vi "SCMP - Main Program v3.vi"() -> ()   [LabVIEW 2014]
doc: "Goodrich Exposure Range: .05microseconds to 798.9ms\n\nLow Gain (110e-/ADU)\nHigh Gain (6.5 e-/ADU)\n\nGA1280J Trigger Modes\n0 : Internally triggered; Internally timed\n1 : Externally triggered; Internally timed\n2 : Externally triggered; Externally timed\n3 : Externally gated; Internally timed\n\nFor list of camera commands\nsee Appendix A in the manual\n\n\nUse this template to build a standard state machine design pattern. Each state executes code and determines which state to transition to. Contrast this design pattern with the User Interface Event Handler pattern, in which code executes in response to user actions. Contrast this design pattern also with the Queued Message Handler pattern, in which each message handling code can queue zero or more new messages.\nNote: This template does not contain the most recent programming guidelines recommended by National Instruments. For a complete, project-based implementation of the Standard State Machine pattern, use the Create Project dialog box instead of this template."
uses:
  Controls/Main Program States.ctl
  <vilib>/Utility/error.llb/DialogType.ctl
  Controls/SCD - Calibration Optics Filter Wheel.ctl
  Controls/SCD - EDT - Emission Line Filter Wheel.ctl
  Controls/CoMP-S Controls/Emission Line Filter Wheel.ctl
  Controls/CoMP-S Controls/Polarization Optics Filter Wheel.ctl
  Controls/Global demo.vi
  Controls/SCD - FITS Cluster.ctl
  AISAS/Controls/focus.ctl
  AISAS/Controls/Diffuser.ctl
  Controls/Globals.vi
  AISAS/Mech/AISAS Mech.lvclass
  c:/mhutar/SCMP/Ancillary/Watlow EZ-ZONE/Public/Watbus.dll
  Ancillary/Watlow EZ-ZONE/Public/Watbus.dll
  Controls/peripherals.ctl
  AISAS/Controls/motor.ctl
  Camera/Camera/Camera.lvclass
  Controls/Cameras select.ctl
  Camera/Andor Neo/Andor.lvclass
  Controls/FITS Data type.ctl
  Controls/Cbk Data type.ctl
  Controls/Cookbook.ctl
  Controls/beaning.ctl
  PI/PI Control.ctl
  AISAS/Controls/Rotation.ctl
panel:
  in  "Comment":string="Test"
  in  "Observer":string="Observer"
  out "Instrument":string
  out "Main Loop":bool=TRUE
  out "Log Loop":bool=TRUE
  out "Program":bool=TRUE
  out "Version":string
  in  "AOI Width 2":i64=2560
  in  "AOI Height 2":i64=2160
  out "Latest Actions":string="\r"
  out "cbk name":string="automated_find_focus_656.cbk"
  out "Main Loop Error":errorcluster={"status"=TRUE, "code"=0, "source"=""}
  in  "Tab Control":T1(tab)
  in  "Live Preview":bool
  in  "Snap Images":bool
  out "Camera T Image Zoom":u32[][](graph)
  out "Histogram Graph 2":T2(graph)
  out "Timestamp 2":timestamp=timestamp(3507746192.5616717 s since 1904-01-01)
  out "Mean ADU 2":u32=7788 format="%.1f"
  out "Sharpness 2":dbl format="%.2f"
  out "Camera FITS file path 2":path
  out "Camera R Image":u32[][](graph)
  in  "PI cam3 (mm)":T3 min=0.1 max=21.0 step=0.1 format="%.1f"
  in  "PI cam2 (mm)":T3 min=0.1 max=27.0 step=0.1 format="%.1f"
  in  "Calibration Optics":T4
  in  "Size":dbl format="%.2f"
  in  "Focus":T5 min=70.0 max=152.0 format="%.2f"
  in  "Andover Filter Wheel":T6
  in  "Calibration Wheel":T7
  in  "Binning":T8
  in  "Save Data to FITS?":bool
  out "Histogram Graph":T2(graph)
  in  "Exposure (s)":dbl=0.02 min=1e-05 max=10.0 step=0.001 format="%_3p"
  out "Timestamp":timestamp=timestamp(3507746192.5616717 s since 1904-01-01)
  in  "PI cam1 (mm)":T3 min=0.1 max=27.0 step=0.1 format="%.1f"
  out "Camera FITS file path":path
  in  "Emission Line Filters":T9
  in  "Set Filter Wheels":bool
  out "Mean ADU":u32=7788 format="%.1f"
  out "Sharpness":dbl format="%.2f"
  in  "Diffuser":T10=enum."In Beam"
  in  "Rotation [deg]":T11 min=0.0 max=360.0 step=1.0 format="%.1f"
  in  "Move AISAS Mechanisms":bool
  in  "Motors":bool=TRUE
  out "Camera Image":u32[][](graph)
  out "Camera T Image":u32[][](graph)
  in  "Wavelength [nm]":dbl=557.0 min=0.0 step=0.01 format="%.2f"
  in  "Cameras":T12
  in  "preset cbk":u16(ring) caption="focus/filter/PIs/texp" items=["530.3nm (Fe XIV)", "587.6nm (He I D3)", "637.5nm (Fe X)", "656.3nm (H-Alpha)", "854.2nm (Ca I)", "1074.7nm (Fe XIII)", "1079.8nm (Fe XIII)", "1083.0nm (He I)"]
  in  "Run Cookbook":bool
  in  "Save Data to FITS?":bool=TRUE
  out "Cookbook":T13=[{"Data Type"=enum."ACQUIRE DATA", "Arg 1"=0.0, "Arg 2"=0.0, "Arg 3"=path "", "Comments"=""}, {"Data Type"=enum."ACQUIRE DATA", "Arg 1"=0.0, "Arg 2"=0.0, "Arg 3"=path "", "Comments"=""}]
  out "FITS Path from Last Recipe Acquiring Data":path
  out "# of Recipes":i16
  out "Selected Cookbook":path
  out "Recipe Files":string[](array[string])
  in  "limit max FPS to:":dbl=10.0 min=0.1 max=49.0 step=1.0 format="%.1g"
  out "Continually Read Log File":string="20160903-07:42:55 Live Preview Images\n20160903-07:44:38 Program Terminated\n20160903-07:45:16 Program Started\n20160903-07:45:18 Snap Single Image\n20160903-07:45:27 Live Preview Images\n20160903-07:46:17 Calibration & Filter wheel position:\t8\t5\n20160903-07:46:35 Live Preview Images\n20160903-07:50:39 Live Preview Images\n20160903-07:51:54 Camera Moved to Positon:-18.00\n20160903-07:51:55 Snap Single Image\n20160903-07:52:37 Loaded Cookbook\tfind_focus_656.cbk\n20160903-07:53:52 Run Cookbook\tfind_focus_656.cbk\n20160903-07:53:52 Recipe#0-exposure-20ms.rcp\n20160903-07:53:52 Recipe#1-fw-656.rcp\n20160903-07:53:54 Recipe#2-cal-open.rcp\n20160903-07:53:56 Recipe#3-move-absolute-neg19.rcp\n20160903-07:53:56 Recipe#4-take_656_focus_image.rcp\n20160903-07:54:02 Recipe#5-move-relative-neg0pt25.rcp\n20160903-07:55:56 Program Started\n20160903-07:56:02 Camera Moved to Positon:-18.00\n20160903-07:56:03 Snap Single Image\n20160903-07:56:35 Camera Moved to Positon:-19.00\n20160903-07:56:37 Snap Single Image\n20160903-07:56:58 Camera Moved to Positon:-20.00\n20160903-07:57:02 Snap Single Image\n20160903-07:57:20 Camera Moved to Positon:-21.00\n20160903-07:57:23 Snap Single Image\n20160903-07:57:36 Camera Moved to Positon:-22.00\n20160903-07:57:37 Snap Single Image\n20160903-07:57:53 Camera Moved to Positon:-25.00\n20160903-07:57:57 Snap Single Image\n20160903-07:58:13 Camera Moved to Positon:-30.00\n20160903-07:58:17 Snap Single Image\n20160903-07:58:43 Camera Moved to Positon:-18.00\n20160903-07:58:44 Snap Single Image\n20160903-07:58:58 Camera Moved to Positon:-17.00\n20160903-07:59:00 Snap Single Image\n20160903-08:00:39 Calibration & Filter wheel position:\t7\t6\n20160903-08:00:48 Snap Single Image\n20160903-08:01:42 Camera Moved to Positon:-65.00\n20160903-08:01:47 Snap Single Image\n20160903-08:02:07 Camera Moved to Positon:-70.00\n20160903-08:02:10 Snap Single Image\n20160903-08:02:51 Camera Moved to Positon:-75.00\n20160903-08:02:53 Snap Single Image\n20160903-08:03:25 Calibration & Filter wheel position:\t7\t7\n20160903-08:03:37 Snap Single Image\n20160903-08:03:55 Camera Moved to Positon:-76.00\n20160903-08:04:01 Snap Single Image\n20160903-08:04:13 Camera Moved to Positon:-77.00\n20160903-08:04:14 Snap Single Image\n20160903-08:04:24 Camera Moved to Positon:-78.00\n20160903-08:04:26 Snap Single Image\n20160903-08:04:38 Camera Moved to Positon:-79.00\n20160903-08:04:39 Snap Single Image\n20160903-08:04:50 Camera Moved to Positon:-83.00\n20160903-08:04:52 Snap Single Image\n20160903-08:05:10 Camera Moved to Positon:-73.00\n20160903-08:05:11 Snap Single Image\n20160903-08:05:22 Camera Moved to Positon:-71.00\n20160903-08:05:24 Snap Single Image\n20160903-08:05:34 Camera Moved to Positon:-69.00\n20160903-08:05:35 Snap Single Image\n20160903-08:05:47 Camera Moved to Positon:-67.00\n20160903-08:05:48 Snap Single Image\n20160903-08:06:13 Calibration & Filter wheel position:\t7\t8\n20160903-08:07:06 Snap Single Image\n20160903-08:07:17 Camera Moved to Positon:-69.00\n20160903-08:07:18 Snap Single Image\n20160903-08:07:28 Camera Moved to Positon:-71.00\n20160903-08:07:30 Snap Single Image\n20160903-08:07:40 Camera Moved to Positon:-73.00\n20160903-08:07:43 Snap Single Image\n20160903-08:07:53 Camera Moved to Positon:-75.00\n20160903-08:07:55 Snap Single Image\n20160903-08:08:04 Camera Moved to Positon:-77.00\n20160903-08:08:06 Snap Single Image\n20160903-08:08:17 Camera Moved to Positon:-79.00\n20160903-08:08:28 Snap Single Image\n20160903-08:08:43 Camera Moved to Positon:-81.00\n20160903-08:08:46 Snap Single Image\n20160903-08:09:05 Calibration & Filter wheel position:\t7\t9\n20160903-08:09:48 Camera Moved to Positon:-100.00\n20160903-08:09:50 Snap Single Image\n20160903-08:10:09 Snap Single Image\n20160903-08:10:26 Camera Moved to Positon:-100.00\n20160903-08:10:35 Camera Moved to Positon:-100.00\n20160903-08:10:37 Snap Single Image\n20160903-08:10:54 Camera Moved to Positon:-100.00\n20160903-08:10:59 Program Terminated\n20160903-08:12:25 Program Started\n20160903-08:12:33 Camera Moved to Positon:-100.00\n20160903-08:12:38 Program Terminated\n20160903-08:13:25 Program Started\n20160903-08:13:30 Camera Moved to Positon:-100.00\n20160903-08:13:37 Program Terminated\n20160903-08:14:12 Program Started\n20160903-08:14:19 Camera Moved to Positon:-100.00\n20160903-08:14:22 Snap Single Image\n20160903-08:14:37 Calibration & Filter wheel position:\t7\t9\n20160903-08:14:45 Snap Single Image\n20160903-08:14:56 Camera Moved to Positon:-105.00\n20160903-08:14:57 Snap Single Image\n20160903-08:15:10 Camera Moved to Positon:-110.00\n20160903-08:15:11 Snap Single Image\n20160903-08:15:23 Camera Moved to Positon:-115.00\n20160903-08:15:27 Snap Single Image\n20160903-08:15:39 Camera Moved to Positon:-120.00\n20160903-08:15:40 Snap Single Image\n20160903-08:15:59 Snap Single Image\n20160903-08:16:10 Camera Moved to Positon:-115.00\n20160903-08:16:11 Snap Single Image\n20160903-08:16:21 Camera Moved to Positon:-110.00\n20160903-08:16:22 Snap Single Image\n20160903-08:16:33 Camera Moved to Positon:-105.00\n20160903-08:16:36 Snap Single Image\n20160903-08:16:49 Camera Moved to Positon:-100.00\n20160903-08:16:51 Snap Single Image\n20160903-08:17:03 Camera Moved to Positon:-95.00\n20160903-08:17:05 Snap Single Image\n20160903-08:17:16 Camera Moved to Positon:-90.00\n20160903-08:17:18 Snap Single Image\n20160903-08:17:46 Camera Moved to Positon:-85.00\n20160903-08:17:49 Snap Single Image\n20160903-08:18:00 Camera Moved to Positon:-80.00\n20160903-08:18:02 Snap Single Image\n20160903-08:18:40 Calibration & Filter wheel position:\t7\t4\n20160903-08:18:59 Camera Moved to Positon:-20.00\n20160903-08:19:11 Snap Single Image\n20160903-08:19:23 Camera Moved to Positon:-18.00\n20160903-08:19:25 Snap Single Image\n20160903-08:19:38 Camera Moved to Positon:-22.00\n20160903-08:19:39 Snap Single Image\n20160903-08:19:51 Camera Moved to Positon:-24.00\n20160903-08:19:52 Snap Single Image\n20160903-08:20:04 Calibration & Filter wheel position:\t7\t3\n20160903-08:20:11 Snap Single Image\n20160903-08:20:22 Camera Moved to Positon:-18.00\n20160903-08:20:24 Snap Single Image\n20160903-08:20:39 Camera Moved to Positon:-16.00\n20160903-08:20:40 Snap Single Image\n20160903-08:20:53 Camera Moved to Positon:-14.00\n20160903-08:20:56 Snap Single Image\n20160903-08:21:06 Camera Moved to Positon:-12.00\n20160903-08:21:07 Snap Single Image\n20160903-08:21:16 Camera Moved to Positon:-10.00\n20160903-08:21:24 Snap Single Image\n20160903-08:21:34 Camera Moved to Positon: -8.00\n20160903-08:21:36 Snap Single Image\n20160903-08:22:12 Camera Moved to Positon: -6.00\n20160903-08:22:21 Snap Single Image\n20160903-08:23:09 Calibration & Filter wheel position:\t7\t1\n20160903-08:23:17 Snap Single Image\n20160903-08:23:27 Camera Moved to Positon: -4.00\n20160903-08:23:29 Snap Single Image\n20160903-08:23:37 Camera Moved to Positon: -2.00\n20160903-08:23:38 Snap Single Image\n20160903-08:23:47 Camera Moved to Positon:  0.00\n20160903-08:23:50 Snap Single Image\n20160903-08:26:00 Camera Moved to Positon:-18.00\n20160903-08:26:44 Program Started\n20160903-08:26:59 Camera Moved to Positon:-18.00\n20160903-08:27:05 Loaded Cookbook\tfind_focus_656.cbk\n20160903-08:27:12 Run Cookbook\tfind_focus_656.cbk\n20160903-08:27:12 Recipe#0-exposure-20ms.rcp\n20160903-08:27:12 Recipe#1-fw-656.rcp\n20160903-08:27:14 Recipe#2-cal-open.rcp\n20160903-08:27:16 Recipe#3-take_656_focus_image.rcp\n20160903-08:29:11 Camera Moved to Positon:-19.00\n20160903-08:29:17 Run Cookbook\tfind_focus_656.cbk\n20160903-08:29:17 Recipe#0-exposure-20ms.rcp\n20160903-08:29:17 Recipe#1-fw-656.rcp\n20160903-08:29:19 Recipe#2-cal-open.rcp\n20160903-08:29:21 Recipe#3-take_656_focus_image.rcp\n20160903-08:29:59 Camera Moved to Positon:-20.00\n20160903-08:30:03 Run Cookbook\tfind_focus_656.cbk\n20160903-08:30:03 Recipe#0-exposure-20ms.rcp\n20160903-08:30:03 Recipe#1-fw-656.rcp\n20160903-08:30:05 Recipe#2-cal-open.rcp\n20160903-08:30:07 Recipe#3-take_656_focus_image.rcp\n20160903-08:30:28 Camera Moved to Positon:-21.00\n20160903-08:30:32 Run Cookbook\tfind_focus_656.cbk\n20160903-08:30:32 Recipe#0-exposure-20ms.rcp\n20160903-08:30:32 Recipe#1-fw-656.rcp\n20160903-08:30:34 Recipe#2-cal-open.rcp\n20160903-08:30:36 Recipe#3-take_656_focus_image.rcp\n20160903-08:31:03 Camera Moved to Positon:-22.00\n20160903-08:31:06 Run Cookbook\tfind_focus_656.cbk\n20160903-08:31:06 Recipe#0-exposure-20ms.rcp\n20160903-08:31:06 Recipe#1-fw-656.rcp\n20160903-08:31:08 Recipe#2-cal-open.rcp\n20160903-08:31:10 Recipe#3-take_656_focus_image.rcp\n20160903-08:31:33 Camera Moved to Positon:-23.00\n20160903-08:31:38 Run Cookbook\tfind_focus_656.cbk\n20160903-08:31:38 Recipe#0-exposure-20ms.rcp\n20160903-08:31:38 Recipe#1-fw-656.rcp\n20160903-08:31:40 Recipe#2-cal-open.rcp\n20160903-08:31:42 Recipe#3-take_656_focus_image.rcp\n20160903-08:32:05 Camera Moved to Positon:-24.00\n20160903-08:32:08 Run Cookbook\tfind_focus_656.cbk\n20160903-08:32:08 Recipe#0-exposure-20ms.rcp\n20160903-08:32:08 Recipe#1-fw-656.rcp\n20160903-08:32:10 Recipe#2-cal-open.rcp\n20160903-08:32:12 Recipe#3-take_656_focus_image.rcp\n20160903-08:32:35 Camera Moved to Positon:-25.00\n20160903-08:32:40 Run Cookbook\tfind_focus_656.cbk\n20160903-08:32:40 Recipe#0-exposure-20ms.rcp\n20160903-08:32:40 Recipe#1-fw-656.rcp\n20160903-08:32:42 Recipe#2-cal-open.rcp\n20160903-08:32:44 Recipe#3-take_656_focus_image.rcp\n20160903-08:33:03 Camera Moved to Positon:-26.00\n20160903-08:33:07 Run Cookbook\tfind_focus_656.cbk\n20160903-08:33:07 Recipe#0-exposure-20ms.rcp\n20160903-08:33:07 Recipe#1-fw-656.rcp\n20160903-08:33:09 Recipe#2-cal-open.rcp\n20160903-08:33:11 Recipe#3-take_656_focus_image.rcp\n20160903-08:33:32 Camera Moved to Positon:-27.00\n20160903-08:33:34 Run Cookbook\tfind_focus_656.cbk\n20160903-08:33:34 Recipe#0-exposure-20ms.rcp\n20160903-08:33:34 Recipe#1-fw-656.rcp\n20160903-08:33:36 Recipe#2-cal-open.rcp\n20160903-08:33:38 Recipe#3-take_656_focus_image.rcp\n20160903-08:34:01 Camera Moved to Positon:-28.00\n20160903-08:34:05 Run Cookbook\tfind_focus_656.cbk\n20160903-08:34:05 Recipe#0-exposure-20ms.rcp\n20160903-08:34:05 Recipe#1-fw-656.rcp\n20160903-08:34:07 Recipe#2-cal-open.rcp\n20160903-08:34:09 Recipe#3-take_656_focus_image.rcp\n20160903-08:36:44 Camera Moved to Positon:-85.00\n20160903-08:36:51 Loaded Cookbook\tfind_focus_1083.cbk\n20160903-08:37:11 Loaded Cookbook\tfind_focus_1083.cbk\n20160903-08:37:20 Run Cookbook\tfind_focus_1083.cbk\n20160903-08:37:20 Recipe#0-exposure-120ms.rcp\n20160903-08:37:20 Recipe#1-fw-1083.rcp\n20160903-08:37:22 Recipe#2-cal-open.rcp\n20160903-08:37:23 Recipe#3-take_1083_focus_image.rcp\n20160903-08:38:05 Camera Moved to Positon:-86.00\n20160903-08:38:11 Run Cookbook\tfind_focus_1083.cbk\n20160903-08:38:11 Recipe#0-exposure-120ms.rcp\n20160903-08:38:11 Recipe#1-fw-1083.rcp\n20160903-08:38:13 Recipe#2-cal-open.rcp\n20160903-08:38:15 Recipe#3-take_1083_focus_image.rcp\n20160903-08:38:39 Camera Moved to Positon:-87.00\n20160903-08:38:43 Run Cookbook\tfind_focus_1083.cbk\n20160903-08:38:43 Recipe#0-exposure-120ms.rcp\n20160903-08:38:43 Recipe#1-fw-1083.rcp\n20160903-08:38:45 Recipe#2-cal-open.rcp\n20160903-08:38:47 Recipe#3-take_1083_focus_image.rcp\n20160903-08:39:05 Camera Moved to Positon:-88.00\n20160903-08:39:09 Run Cookbook\tfind_focus_1083.cbk\n20160903-08:39:10 Recipe#0-exposure-120ms.rcp\n20160903-08:39:10 Recipe#1-fw-1083.rcp\n20160903-08:39:12 Recipe#2-cal-open.rcp\n20160903-08:39:13 Recipe#3-take_1083_focus_image.rcp\n20160903-08:43:45 Snap Single Image\n20160903-08:43:56 Run Cookbook\tfind_focus_1083.cbk\n20160903-08:43:56 Recipe#0-exposure-120ms.rcp\n20160903-08:43:56 Recipe#1-fw-1083.rcp\n20160903-08:43:58 Recipe#2-cal-open.rcp\n20160903-08:44:00 Recipe#3-take_1083_focus_image.rcp\n20160903-08:44:24 Camera Moved to Positon:-90.00\n20160903-08:44:32 Camera Moved to Positon:-89.00\n20160903-08:44:36 Run Cookbook\tfind_focus_1083.cbk\n20160903-08:44:36 Recipe#0-exposure-120ms.rcp\n20160903-08:44:36 Recipe#1-fw-1083.rcp\n20160903-08:44:38 Recipe#2-cal-open.rcp\n20160903-08:44:40 Recipe#3-take_1083_focus_image.rcp\n20160903-08:45:03 Camera Moved to Positon:-90.00\n20160903-08:45:11 Run Cookbook\tfind_focus_1083.cbk\n20160903-08:45:12 Recipe#0-exposure-120ms.rcp\n20160903-08:45:12 Recipe#1-fw-1083.rcp\n20160903-08:45:14 Recipe#2-cal-open.rcp\n20160903-08:45:15 Recipe#3-take_1083_focus_image.rcp\n20160903-08:45:38 Camera Moved to Positon:-91.00\n20160903-08:45:41 Run Cookbook\tfind_focus_1083.cbk\n20160903-08:45:41 Recipe#0-exposure-120ms.rcp\n20160903-08:45:42 Recipe#1-fw-1083.rcp\n20160903-08:45:43 Recipe#2-cal-open.rcp\n20160903-08:45:45 Recipe#3-take_1083_focus_image.rcp\n20160903-08:46:07 Camera Moved to Positon:-92.00\n20160903-08:46:12 Run Cookbook\tfind_focus_1083.cbk\n20160903-08:46:12 Recipe#0-exposure-120ms.rcp\n20160903-08:46:12 Recipe#1-fw-1083.rcp\n20160903-08:46:14 Recipe#2-cal-open.rcp\n20160903-08:46:16 Recipe#3-take_1083_focus_image.rcp\n20160903-08:46:53 Camera Moved to Positon:-93.00\n20160903-08:46:56 Run Cookbook\tfind_focus_1083.cbk\n20160903-08:46:56 Recipe#0-exposure-120ms.rcp\n20160903-08:46:56 Recipe#1-fw-1083.rcp\n20160903-08:46:58 Recipe#2-cal-open.rcp\n20160903-08:47:00 Recipe#3-take_1083_focus_image.rcp\n20160903-08:48:13 Calibration & Filter wheel position:\t7\t3\n20160903-08:51:11 Camera Moved to Positon:-10.00\n20160903-08:51:19 Camera Moved to Positon: -5.00\n20160903-08:51:20 Live Preview Images\n20160903-08:51:43 Loaded Cookbook\tfind_focus_589.cbk\n20160903-08:52:08 Loaded Cookbook\tfocus-656.cbk\n20160903-08:52:09 Run Cookbook\tfocus-656.cbk\n20160903-08:52:09 Recipe#0-fw-656.rcp\n20160903-08:52:11 Recipe#1-cal-clear.rcp\n20160903-08:52:13 Recipe#2-exposure-200ms.rcp\n20160903-08:52:13 Recipe#3-focus-656.rcp\n20160903-08:52:24 Program Started\n20160903-08:52:33 Loaded Cookbook\tfocus-656.cbk\n20160903-08:52:40 Camera Moved to Positon: -5.00\n20160903-08:52:46 Loaded Cookbook\tfind_focus_589.cbk\n20160903-08:52:48 Run Cookbook\tfind_focus_589.cbk\n20160903-08:52:48 Recipe#0-exposure-20ms.rcp\n20160903-08:52:48 Recipe#1-fw-589.rcp\n20160903-08:52:50 Recipe#2-cal-open.rcp\n20160903-08:52:52 Recipe#3-take_589_focus_image.rcp\n20160903-08:54:55 Run Cookbook\tfind_focus_589.cbk\n20160903-08:54:55 Recipe#0-exposure-20ms.rcp\n20160903-08:54:56 Recipe#1-fw-589.rcp\n20160903-08:54:57 Recipe#2-cal-open.rcp\n20160903-08:54:59 Recipe#3-take_589_focus_image.rcp\n20160903-08:55:19 Live Preview Images\n20160903-08:56:01 Camera Moved to Positon: -6.00\n20160903-08:56:04 Run Cookbook\tfind_focus_589.cbk\n20160903-08:56:04 Recipe#0-exposure-20ms.rcp\n20160903-08:56:04 Recipe#1-fw-589.rcp\n20160903-08:56:06 Recipe#2-cal-open.rcp\n20160903-08:56:08 Recipe#3-take_589_focus_image.rcp\n20160903-08:56:40 Camera Moved to Positon: -7.00\n20160903-08:58:30 Run Cookbook\tfind_focus_589.cbk\n20160903-08:58:30 Recipe#0-exposure-20ms.rcp\n20160903-08:58:30 Recipe#1-fw-589.rcp\n20160903-08:58:32 Recipe#2-cal-open.rcp\n20160903-08:58:34 Recipe#3-take_589_focus_image.rcp\n20160903-08:59:22 Camera Moved to Positon: -8.00\n20160903-09:14:18 Program Terminated\n20160903-09:40:55 Program Started\n20160903-09:44:03 Loaded Cookbook\tautomated_find_focus_656.cbk\n20160903-09:44:43 Loaded Cookbook\tautomated_find_focus_656.cbk\n20160903-09:44:57 Run Cookbook\tautomated_find_focus_656.cbk\n20160903-09:44:57 Recipe#0-exposure-20ms.rcp\n20160903-09:44:57 Recipe#1-fw-656.rcp\n20160903-09:44:59 Recipe#2-cal-open.rcp\n20160903-09:45:01 Recipe#3-move-absolute-neg15.rcp\n20160903-09:45:02 Recipe#4-take_656_focus_image.rcp\n20160903-09:45:16 Recipe#5-move-relative-neg0pt25.rcp\n20160903-09:45:17 Recipe#6-take_656_focus_image.rcp\n20160903-09:45:31 Recipe#7-move-relative-neg0pt25.rcp\n20160903-09:45:32 Recipe#8-take_656_focus_image.rcp\n20160903-09:45:46 Recipe#9-move-relative-neg0pt25.rcp\n20160903-09:45:47 Recipe#10-take_656_focus_image.rcp\n20160903-09:46:01 Recipe#11-move-relative-neg0pt25.rcp\n20160903-09:46:02 Recipe#12-take_656_focus_image.rcp\n20160903-09:46:17 Recipe#13-move-relative-neg0pt25.rcp\n20160903-09:46:18 Recipe#14-take_656_focus_image.rcp\n20160903-09:46:32 Recipe#15-move-relative-neg0pt25.rcp\n20160903-09:46:33 Recipe#16-take_656_focus_image.rcp\n20160903-09:46:47 Recipe#17-move-relative-neg0pt25.rcp\n20160903-09:46:48 Recipe#18-take_656_focus_image.rcp\n20160903-09:47:02 Recipe#19-move-relative-neg0pt25.rcp\n20160903-09:47:03 Recipe#20-take_656_focus_image.rcp\n20160903-09:47:17 Recipe#21-move-relative-neg0pt25.rcp\n20160903-09:47:17 Recipe#22-take_656_focus_image.rcp\n20160903-09:47:32 Recipe#23-move-relative-neg0pt25.rcp\n20160903-09:47:32 Recipe#24-take_656_focus_image.rcp\n20160903-09:47:46 Recipe#25-move-relative-neg0pt25.rcp\n20160903-09:47:47 Recipe#26-take_656_focus_image.rcp\n20160903-09:48:02 Recipe#27-move-relative-neg0pt25.rcp\n20160903-09:48:03 Recipe#28-take_656_focus_image.rcp\n20160903-09:48:17 Recipe#29-move-relative-neg0pt25.rcp\n20160903-09:48:17 Recipe#30-take_656_focus_image.rcp\n20160903-09:48:32 Recipe#31-move-relative-neg0pt25.rcp\n20160903-09:48:33 Recipe#32-take_656_focus_image.rcp\n20160903-09:48:49 Recipe#33-move-relative-neg0pt25.rcp\n20160903-09:48:49 Recipe#34-take_656_focus_image.rcp\n20160903-09:49:05 Recipe#35-move-relative-neg0pt25.rcp\n20160903-09:49:06 Recipe#36-take_656_focus_image.rcp\n20160903-09:49:23 Recipe#37-move-relative-neg0pt25.rcp\n20160903-09:49:24 Recipe#38-take_656_focus_image.rcp\n20160903-09:49:41 Recipe#39-move-relative-neg0pt25.rcp\n20160903-09:49:42 Recipe#40-take_656_focus_image.rcp\n20160903-09:50:01 Recipe#41-move-relative-neg0pt25.rcp\n20160903-09:50:01 Recipe#42-take_656_focus_image.rcp\n20160903-09:50:20 Recipe#43-move-relative-neg0pt25.rcp\n20160903-09:50:21 Recipe#44-take_656_focus_image.rcp\n20160903-09:54:36 Loaded Cookbook\tautomated_find_focus_656.cbk\n20160903-09:54:47 Loaded Cookbook\tautomated_find_focus_656.cbk\n20160903-09:55:40 Loaded Cookbook\tautomated_find_focus_656.cbk\n20160903-09:55:54 Run Cookbook\tautomated_find_focus_656.cbk\n20160903-09:55:54 Recipe#0-exposure-40ms.rcp\n20160903-09:55:54 Recipe#1-fw-656.rcp\n20160903-09:55:56 Recipe#2-cal-open.rcp\n20160903-09:55:58 Recipe#3-move-absolute-neg15.rcp\n20160903-09:55:59 Recipe#4-take_656_focus_image.rcp\n20160903-09:56:06 Recipe#5-move-relative-neg0pt5.rcp\n20160903-09:56:07 Recipe#6-take_656_focus_image.rcp\n20160903-09:56:14 Recipe#7-move-relative-neg0pt5.rcp\n20160903-09:56:15 Recipe#8-take_656_focus_image.rcp\n20160903-09:56:22 Recipe#9-move-relative-neg0pt5.rcp\n20160903-09:56:22 Recipe#10-take_656_focus_image.rcp\n20160903-09:56:29 Recipe#11-move-relative-neg0pt5.rcp\n20160903-09:56:30 Recipe#12-take_656_focus_image.rcp\n20160903-09:56:37 Recipe#13-move-relative-neg0pt5.rcp\n20160903-09:56:38 Recipe#14-take_656_focus_image.rcp\n20160903-09:56:45 Recipe#15-move-relative-neg0pt5.rcp\n20160903-09:56:45 Recipe#16-take_656_focus_image.rcp\n20160903-09:56:52 Recipe#17-move-relative-neg0pt5.rcp\n20160903-09:56:53 Recipe#18-take_656_focus_image.rcp\n20160903-09:57:00 Recipe#19-move-relative-neg0pt5.rcp\n20160903-09:57:01 Recipe#20-take_656_focus_image.rcp\n20160903-09:57:08 Recipe#21-move-relative-neg0pt5.rcp\n20160903-09:57:09 Recipe#22-take_656_focus_image.rcp\n20160903-09:57:16 Recipe#23-move-relative-neg0pt5.rcp\n20160903-09:57:16 Recipe#24-take_656_focus_image.rcp\n20160903-09:57:23 Recipe#25-move-relative-neg0pt5.rcp\n20160903-09:57:24 Recipe#26-take_656_focus_image.rcp\n20160903-09:57:31 Recipe#27-move-relative-neg0pt5.rcp\n20160903-09:57:32 Recipe#28-take_656_focus_image.rcp\n20160903-09:57:39 Recipe#29-move-relative-neg0pt5.rcp\n20160903-09:57:40 Recipe#30-take_656_focus_image.rcp\n20160903-09:57:47 Recipe#31-move-relative-neg0pt5.rcp\n20160903-09:57:48 Recipe#32-take_656_focus_image.rcp\n20160903-09:57:55 Recipe#33-move-relative-neg0pt5.rcp\n20160903-09:57:56 Recipe#34-take_656_focus_image.rcp\n20160903-09:58:03 Recipe#35-move-relative-neg0pt5.rcp\n20160903-09:58:03 Recipe#36-take_656_focus_image.rcp\n20160903-09:58:10 Recipe#37-move-relative-neg0pt5.rcp\n20160903-09:58:11 Recipe#38-take_656_focus_image.rcp\n20160903-09:58:18 Recipe#39-move-relative-neg0pt5.rcp\n20160903-09:58:19 Recipe#40-take_656_focus_image.rcp\n20160903-09:58:26 Recipe#41-move-relative-neg0pt5.rcp\n20160903-09:58:27 Recipe#42-take_656_focus_image.rcp\n20160903-09:58:34 Recipe#43-move-relative-neg0pt5.rcp\n20160903-09:58:35 Recipe#44-take_656_focus_image.rcp\n20160903-10:46:33 Program Terminated\n20160903-12:25:32 Program Started\n20160903-12:26:22 Program Terminated\n20160903-12:45:45 Program Started\n20160903-12:45:56 Program Terminated\n20160903-12:49:12 Program Started\n20160903-12:49:15 Loaded Cookbook\tautomated_find_focus_656.cbk\n20160903-12:49:24 Run Cookbook\tautomated_find_focus_656.cbk\n20160903-12:49:25 Recipe#0-exposure-40ms.rcp\n20160903-12:49:25 Recipe#1-fw-656.rcp\n20160903-12:49:26 Recipe#2-cal-open.rcp\n20160903-12:49:28 Recipe#3-move-absolute-neg15.rcp\n20160903-12:49:29 Recipe#4-take_656_focus_image.rcp\n20160903-12:49:32 Recipe#5-move-relative-neg0pt5.rcp\n20160903-12:49:33 Recipe#6-take_656_focus_image.rcp\n20160903-12:49:36 Recipe#7-move-relative-neg0pt5.rcp\n20160903-12:49:36 Recipe#8-take_656_focus_image.rcp\n20160903-12:49:39 Recipe#9-move-relative-neg0pt5.rcp\n20160903-12:49:40 Recipe#10-take_656_focus_image.rcp\n20160903-12:49:43 Recipe#11-move-relative-neg0pt5.rcp\n20160903-12:49:43 Recipe#12-take_656_focus_image.rcp\n20160903-12:49:46 Recipe#13-move-relative-neg0pt5.rcp\n20160903-12:49:47 Recipe#14-take_656_focus_image.rcp\n20160903-12:49:49 Recipe#15-move-relative-neg0pt5.rcp\n20160903-12:49:50 Recipe#16-take_656_focus_image.rcp\n20160903-12:49:53 Recipe#17-move-relative-neg0pt5.rcp\n20160903-12:49:53 Recipe#18-take_656_focus_image.rcp\n20160903-12:49:56 Recipe#19-move-relative-neg0pt5.rcp\n20160903-12:49:57 Recipe#20-take_656_focus_image.rcp\n20160903-12:49:59 Recipe#21-move-relative-neg0pt5.rcp\n20160903-12:50:00 Recipe#22-take_656_focus_image.rcp\n20160903-12:50:03 Recipe#23-move-relative-neg0pt5.rcp\n20160903-12:50:04 Recipe#24-take_656_focus_image.rcp\n20160903-12:50:06 Recipe#25-move-relative-neg0pt5.rcp\n20160903-12:50:07 Recipe#26-take_656_focus_image.rcp\n20160903-12:50:10 Recipe#27-move-relative-neg0pt5.rcp\n20160903-12:50:10 Recipe#28-take_656_focus_image.rcp\n20160903-12:50:13 Recipe#29-move-relative-neg0pt5.rcp\n20160903-12:50:14 Recipe#30-take_656_focus_image.rcp\n20160903-12:50:16 Recipe#31-move-relative-neg0pt5.rcp\n20160903-12:50:17 Recipe#32-take_656_focus_image.rcp\n20160903-12:50:20 Recipe#33-move-relative-neg0pt5.rcp\n20160903-12:50:20 Recipe#34-take_656_focus_image.rcp\n20160903-12:50:23 Recipe#35-move-relative-neg0pt5.rcp\n20160903-12:50:24 Recipe#36-take_656_focus_image.rcp\n20160903-12:50:26 Recipe#37-move-relative-neg0pt5.rcp\n20160903-12:50:27 Recipe#38-take_656_focus_image.rcp\n20160903-12:50:30 Recipe#39-move-relative-neg0pt5.rcp\n20160903-12:50:31 Recipe#40-take_656_focus_image.rcp\n20160903-12:50:33 Recipe#41-move-relative-neg0pt5.rcp\n20160903-12:50:34 Recipe#42-take_656_focus_image.rcp\n20160903-12:50:37 Recipe#43-move-relative-neg0pt5.rcp\n20160903-12:50:37 Recipe#44-take_656_focus_image.rcp\n20160903-13:54:17 Program Terminated\n20160903-14:07:18 Program Started\n20160903-14:08:12 Program Terminated\n20160903-14:20:46 Program Started\n20160903-14:22:56 Program Terminated\n20160903-14:23:20 Program Started\n20160903-14:25:03 Program Terminated\n20160903-14:31:16 Program Started\n20160903-14:32:59 Program Terminated\n20160903-14:33:26 Program Started\n20160903-14:35:01 Program Terminated\n20160903-14:36:43 Program Started\n20160903-14:38:01 Program Terminated\n20160903-14:39:22 Program Started\n20160903-14:39:47 Program Terminated\n20160903-14:40:22 Program Started\n20160903-14:41:59 Program Terminated\n20160903-15:07:40 Program Started\n20160903-15:10:18 Program Terminated\n20160903-15:19:59 Program Started\n20160903-15:20:17 Program Terminated\n20160903-15:20:43 Program Started\n20160903-15:20:43 Program Terminated\n20160903-15:21:33 Program Started\n20160903-15:22:45 Program Terminated\n20160903-15:24:43 Program Started\n20160903-15:26:40 Program Terminated\n20160903-15:29:07 Program Started\n20160903-15:29:52 Loaded Cookbook\tautomated_find_focus_656.cbk\n20160903-15:30:08 Loaded Cookbook\tautomated_find_focus_656.cbk\n"
  out "min Cookbook Exposure [s]":dbl=200.0 format="%#_3p"
  out "Today's SCMP Log File":path
  out "Cookbook Comments":string
  in  "Mod/Seq":bool
  in  "Load Cookbook":bool
  in  "Enable Data Logging":bool=TRUE
  out "Today's SCMP Eng  File":path
  out "Air around \nprefilter wheel [C]":sgl(graph)
  out "Lyot Filter Temp [C]":dbl(graph)
  out "Air around Camera [C]":sgl(graph)
  out "Air around Lyot Filter [C]":dbl(graph)
  out "Eng Data Error":errorcluster={"status"=TRUE, "code"=0, "source"=""}
  out "Camera 1 Temp [C}":dbl(graph)=-21.03
  out "Camera 2 Temp [C}":dbl(graph)=-21.03
  in  "Andor Adv Settings":bool
  out "FITS Header":T15={"Wavelength (nm)"=530.15, "Exposure (s)"=0.05, "Tuning Delay (ms)"=1000.0, "Beam Type (-1/1)"=1.0, "Tuning Voltages"=[1.111, 2.222, 3.333, 4.444], "Observer"="observer", "Light Shapping Diffuser"=enum."In Beam", "Comment"="", "Data Type"=9, "Mod Cycles"=0, "SCD Calibration Optics"=enum."1 - Polarizer @0, I+Q", "SCD Emission Line Filter"=enum."1-557.6nm", "Cookbook"="", "COMP-S Calibration Wheel"=enum."Dark", "COMP-S Andover Filter Wheel"=enum."530.3nm/HWB 0.34nm (Fe XIV)", "FOV Rotation (deg)"=66.0, "Objective Lens Position (mm)"=0.0, "Occulter size"=0.0, "Time End"=timestamp(3382374145.421875 s since 1904-01-01), "Acc Exposure (s)"=0.0, "Time Stamp Array"=[], "Camera Serial Number"=[], "Camera Temp"=[], "Camera PI (mm)"=[], "Time Start"=timestamp(3382374145.421875 s since 1904-01-01), "Peripherals"={"ILX controler"=FALSE, "Zone temperatures"=FALSE, "Andor"=FALSE, "Andor 2"=FALSE, "PI Stages"=FALSE, "AISAS mechanisms"=FALSE, "AISAS Mech.lvclass"=refnum, "Zone temp ref"=variant, "FWs"=FALSE}, "FITS paths"=[], "Cameras"=enum."Andor", "load preset cbk"=FALSE, "periodic check count"=0, "COMP-S Calibration Wheel 2"=enum."Dark", "Calib"=enum."Dark", "Abso Aperture"=40.0, "Nominal Aperture"=196.0} {"Nominal Aperture" format="%.1f"; "Abso Aperture" format="%.1f"; "Camera PI (mm)" format="%_3g"; "Acc Exposure (s)" format="%^.3g"; "Occulter size" format="%.2f"; "Objective Lens Position (mm)" min=70.0 max=152.0 format="%.2f"; "FOV Rotation (deg)" format="%.1f"; "Data Type" items=["LIVE", "DARK", "FLAT", "CALI", "OBSE", "ABSO", "AURE", "TARG", "OBJE", "HOLE", "OREX", "THRO", "CHIP"]; "Exposure (s)" format="%^.3g"; "Wavelength (nm)" format="%_6g"}
  in  "Andor Adv Settings":bool
  in  "Stop":bool=TRUE
  # "Camera Settings"
  # "Filter Wheels"
  # "Coronograph+Instrument Setup"
  # "AISAS mechanisms"
  # "Occulter"
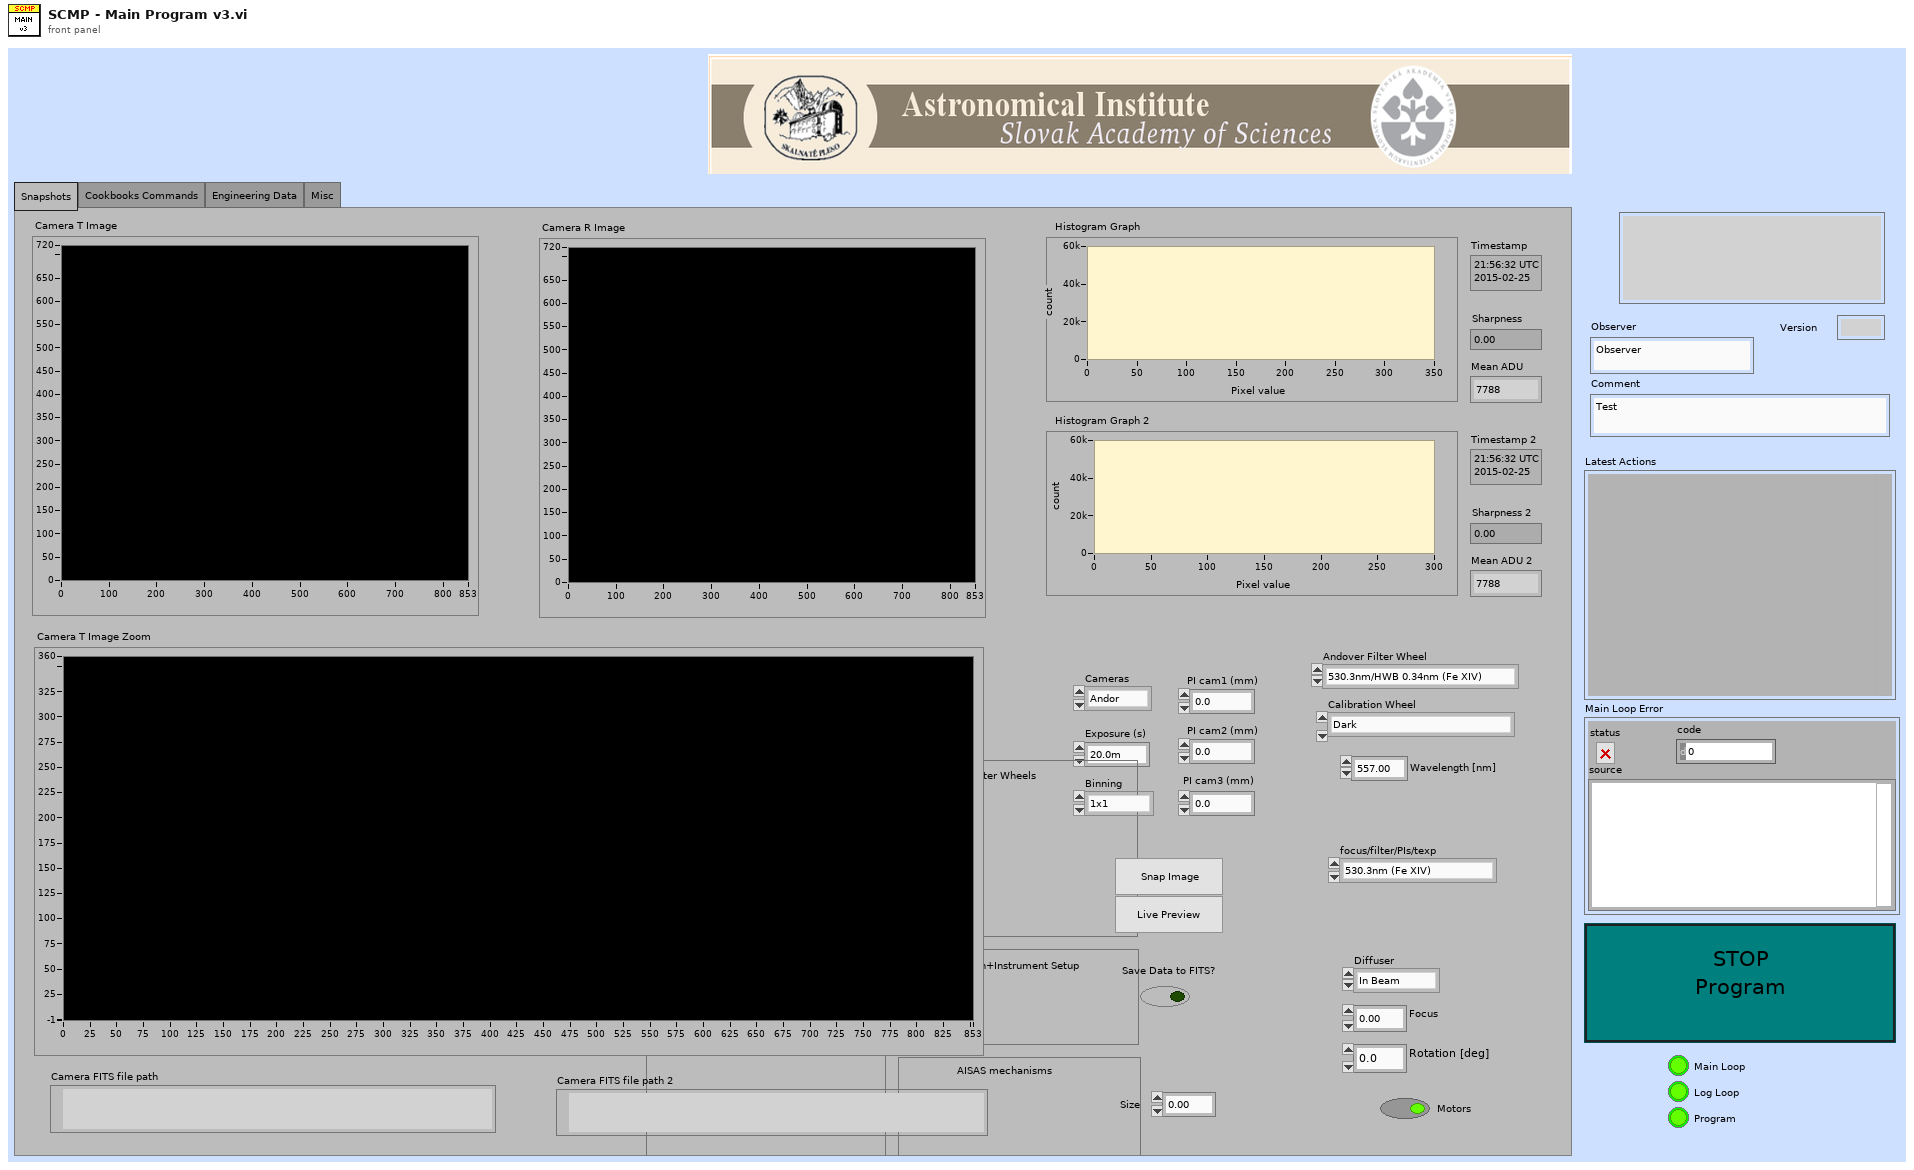
[diagram p1: front panel]
types:
  T1 = enum32{"Snapshots", "Cookbooks Commands", "Engineering Data", "Misc"}
  T2 = cluster{"X Values":dbl[], "Histogram: h(x)":i32[]}
  T3 = typedef "PI Control.ctl" = dbl
  T4 = typedef "SCD - Calibration Optics Filter Wheel.ctl" = enum16{"1 - Polarizer @0, I+Q", "2 - Polarizer @90, I-Q", "3 - Polarizer @45, I+U", "4 - Polarizer @135, I-U", "5 - Polarizer @0, Retarder @45, I+V", "6 - Polarizer @0, Retarder @135, I-V", "7 - Dark", "8 - Clear", "9 - N/A"}
  T5 = typedef "focus.ctl" = dbl
  T6 = typedef "Emission Line Filter Wheel.ctl" = enum16{"530.3nm/HWB 0.34nm (Fe XIV)", "587.6nm/HBW 0.44nm (He I D3)", "637.5nm/HBW 0.53nm (Fe X)", "656.3nm/HBW 0.57nm (H-Alpha)", "789.2nm/HBW 0.85nm (Fe XI)", "854.2nm/HBW 1.01nm (Ca I)", "1074.7nm/HBW 2.34nm (Fe XIII)", "1079.8nm/HBW 1.64nm (Fe XIII)", "1083.0nm/HBW 1.66nm (He I)"}
  T7 = typedef "Polarization Optics Filter Wheel.ctl" = enum16{"Dark", "Clear", "Exchange Lens", "Polarizer @0, I+Q", "Polarizer @90, I-Q", "Polarizer @45, I+U", "Polarizer @135, I-U", "Polarizer @0, Retarder @45, I+V", "Polarizer @0, Retarder @135, I-V"}
  T8 = typedef "beaning.ctl" = enum16{"1x1", "2x2", "3x3", "4x4", "8x8"}
  T9 = typedef "SCD - EDT - Emission Line Filter Wheel.ctl" = enum16{"1-557.6nm", "2-587.6nm", "3-589.6nm", "4-630.2nm", "5-656.4nm", "6-849.8nm", "7-854.2nm", "8-866.2nm", "9-1083.0nm"}
  T10 = typedef "Diffuser.ctl" = enum16{"Out of Beam", "In Beam"}
  T11 = typedef "Rotation.ctl" = dbl
  T12 = typedef "Cameras select.ctl" = enum16{"Andor", "GDR"}
  T13 = typedef "Cookbook.ctl" = cluster{"Data Type":T14, "Arg 1":sgl, "Arg 2":sgl, "Arg 3":path, "Comments":string}[]
  T14 = typedef "Cbk Data type.ctl" = enum32{"ACQUIRE DATA", "SET DIFFUSER", "CAL-FW", "WAVELENGTH-FW", "INSTR. ROTATION", "SET FOCUS", "DATATYPE", "SET EXPOSURE", "CBK COMMENTS", "MOVE-PI", "MOVE-PI2", "MOVE-PI3", "DWELL TIME", "BINNING"}
  T15 = typedef "SCD - FITS Cluster.ctl" = cluster{"Wavelength (nm)":dbl, "Exposure (s)":dbl, "Tuning Delay (ms)":dbl, "Beam Type (-1/1)":dbl, "Tuning Voltages":dbl[], "Observer":string, "Light Shapping Diffuser":T10, "Comment":string, "Data Type":u16, "Mod Cycles":u16, "SCD Calibration Optics":T4, "SCD Emission Line Filter":T9, "Cookbook":string, "COMP-S Calibration Wheel":T7, "COMP-S Andover Filter Wheel":T6, "FOV Rotation (deg)":dbl, "Objective Lens Position (mm)":T5, "Occulter size":dbl, "Time End":timestamp, "Acc Exposure (s)":dbl, "Time Stamp Array":timestamp[], "Camera Serial Number":string[], "Camera Temp":dbl[], "Camera PI (mm)":dbl[], "Time Start":timestamp, "Peripherals":T16, "FITS paths":path[], "Cameras":T12, "load preset cbk":bool, "periodic check count":i32, "COMP-S Calibration Wheel 2":T7, "Calib":enum16{"Dark", "Flat"}, "Abso Aperture":dbl, "Nominal Aperture":dbl}
  T16 = typedef "peripherals.ctl" = cluster{"ILX controler":bool, "Zone temperatures":bool, "Andor":bool, "Andor 2":bool, "PI Stages":bool, "AISAS mechanisms":bool, "AISAS Mech.lvclass":refnum<class "AISAS Mech.lvclass">, "Zone temp ref":variant, "FWs":bool}
  T17 = typedef "Main Program States.ctl" = enum16{"Initialize", "Wait for Event", "Periodic Check", "Update UI", "Update Camera UI", "Load Cookbook", "Run Cookbook", "Snap Images", "Live Preview", "Set Filter Wheel", "Set Calibration Wheel", "AISAS Motors on/off", "AISAS Move", "Move AISAS Mechanisms", "Stop", "Change Camera Exposure", "Change Camera Stage Position", "Set Camera AOI", "Andor Adv Settings", "Update Image", "Run Dark", "Calib acq", "Process Calib"}
  T18 = typedef "SCD - FITS Cluster.ctl" = cluster{"Wavelength (nm)":dbl, "Exposure (s)":dbl, "Tuning Delay (ms)":dbl, "Beam Type (-1/1)":dbl, "Tuning Voltages":dbl[], "Observer":string, "Light Shapping Diffuser":T10, "Comment":string, "Data Type":T19, "Mod Cycles":u16, "SCD Calibration Optics":T4, "SCD Emission Line Filter":T9, "Cookbook":string, "COMP-S Calibration Wheel":T7, "COMP-S Andover Filter Wheel":T6, "FOV Rotation (deg)":dbl, "Objective Lens Position (mm)":T5, "Occulter size":dbl, "Time End":timestamp, "Acc Exposure (s)":dbl, "Time Stamp Array":timestamp[], "Camera Serial Number":string[], "Camera Temp":dbl[], "Camera PI (mm)":dbl[], "Time Start":timestamp, "Peripherals":T16, "FITS paths":path[], "Cameras":T12, "load preset cbk":bool, "periodic check count":i32, "COMP-S Calibration Wheel 2":T7, "Calib":enum16{"Dark", "Flat"}, "Abso Aperture":dbl, "Nominal Aperture":dbl, "Pointer IP":string}
  T19 = typedef "FITS Data type.ctl" = enum16{"LIVE", "DARK", "FLAT", "CALI", "OBSE", "ABSO", "AURE", "TARG", "OBJE", "HOLE", "OREX", "THRO", "CHIP"}
  T20 = enum8{"Enabled", "Disabled", "Disabled and Grayed Out"}
  T21 = enum32{"Invalid", "Standard", "Closed", "Hidden", "Minimized", "Maximized"}
  T22 = typedef "motor.ctl" = enum32{"Rotation", "Diffuser ", "Focus"}
  T23 = enum16{"Emission Line Filters", "Calibration Polarizers"}
  T24 = typedef "DialogType.ctl" = u16
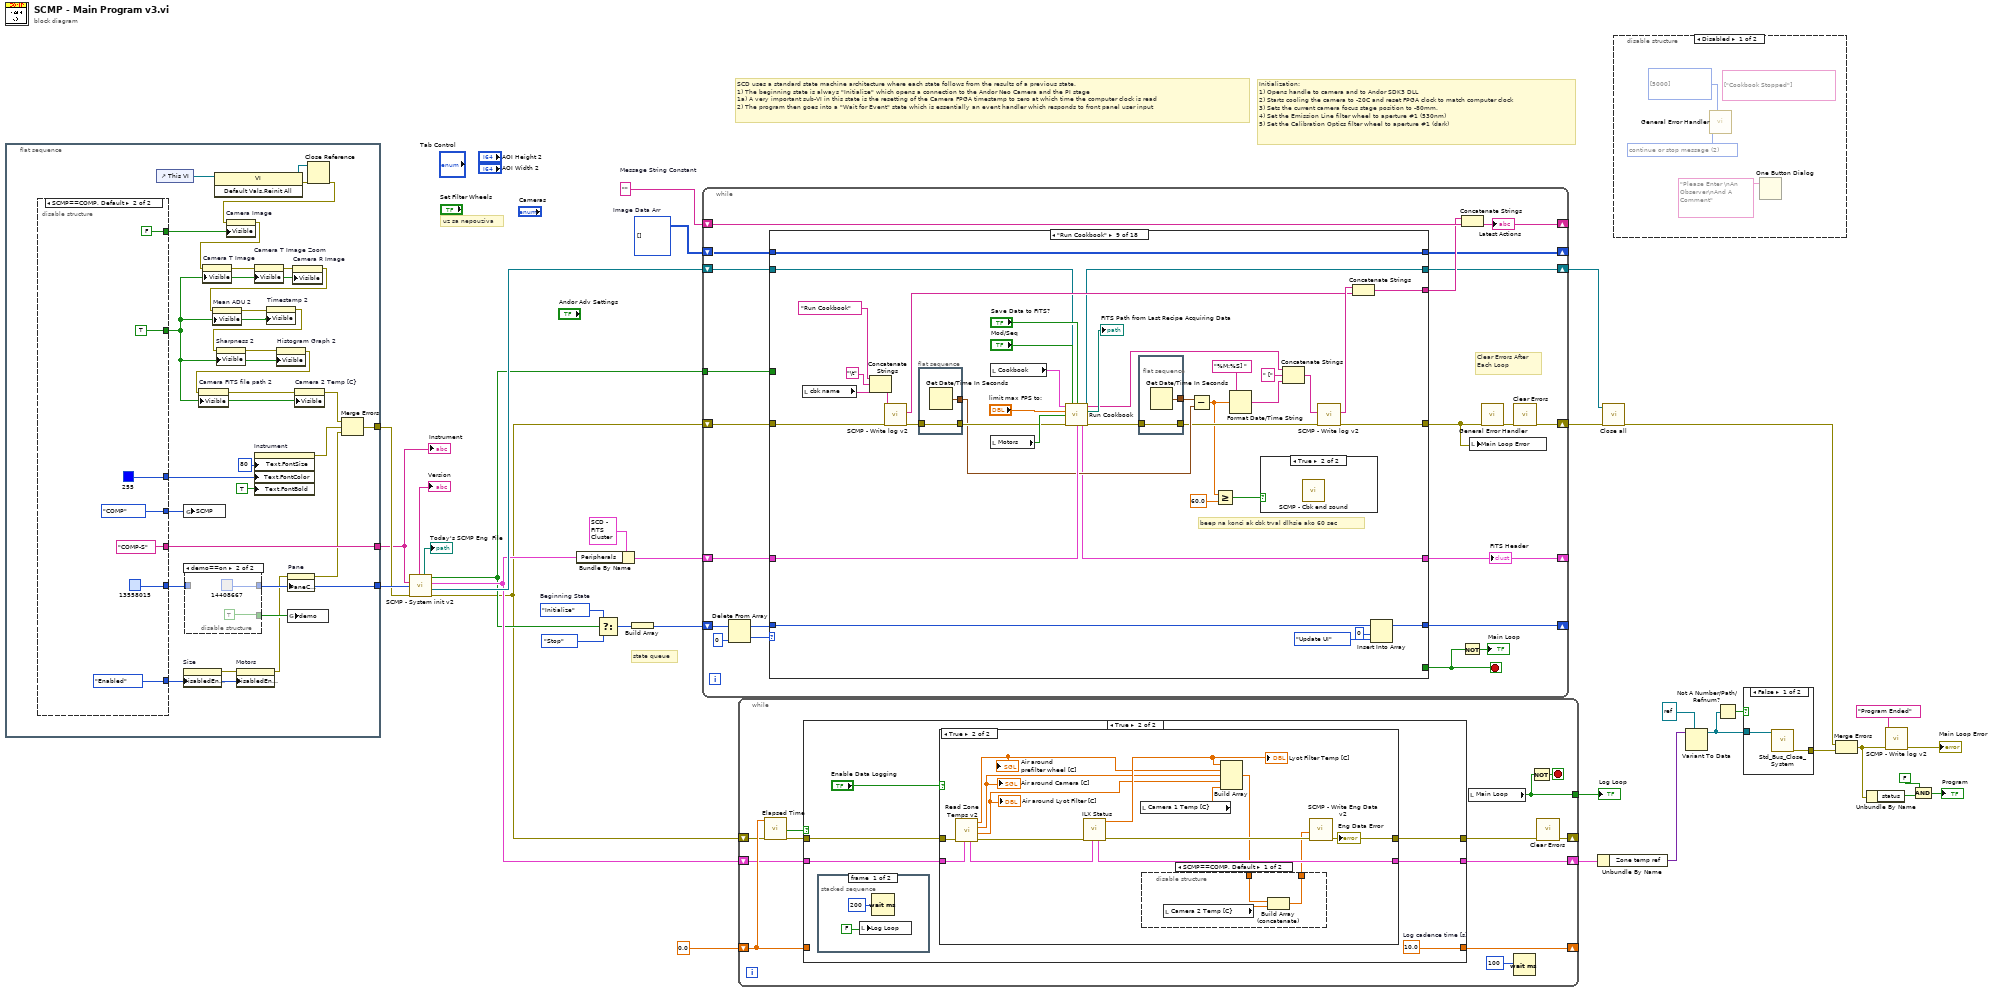
[diagram p0: block diagram]
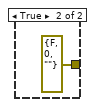
[diagram p2: hidden frame]
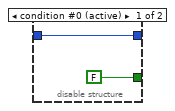
[diagram p3: hidden frame]
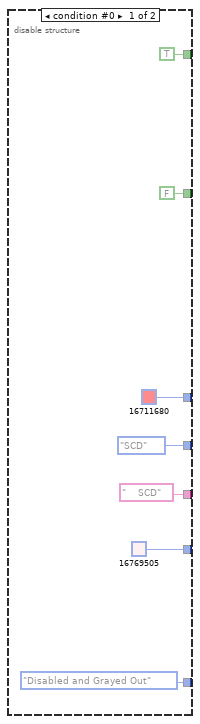
[diagram p4: hidden frame]
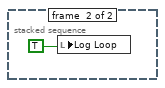
[diagram p7: hidden frame]
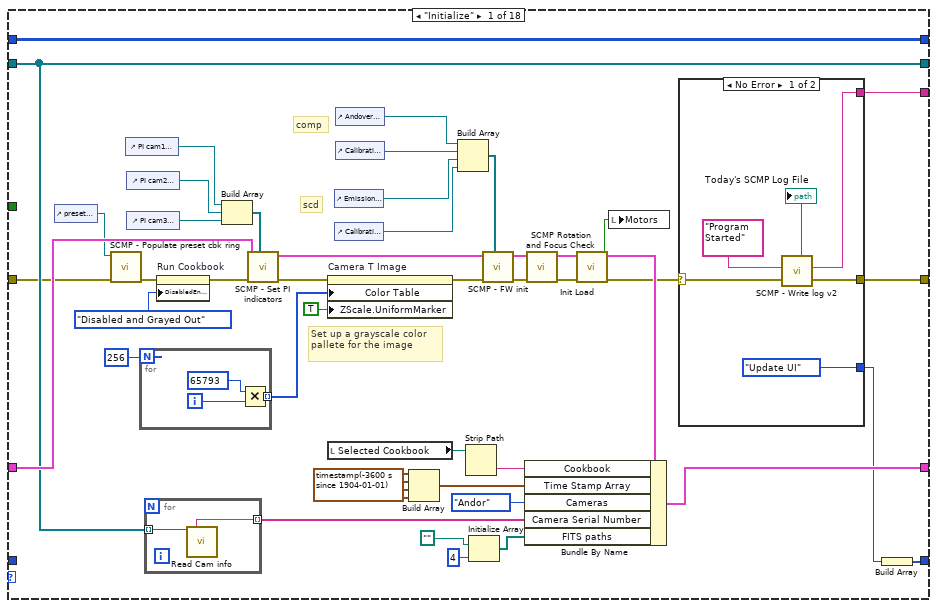
[diagram p10: hidden frame]
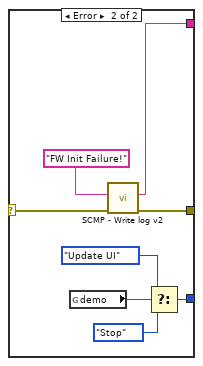
[diagram p11: hidden frame]
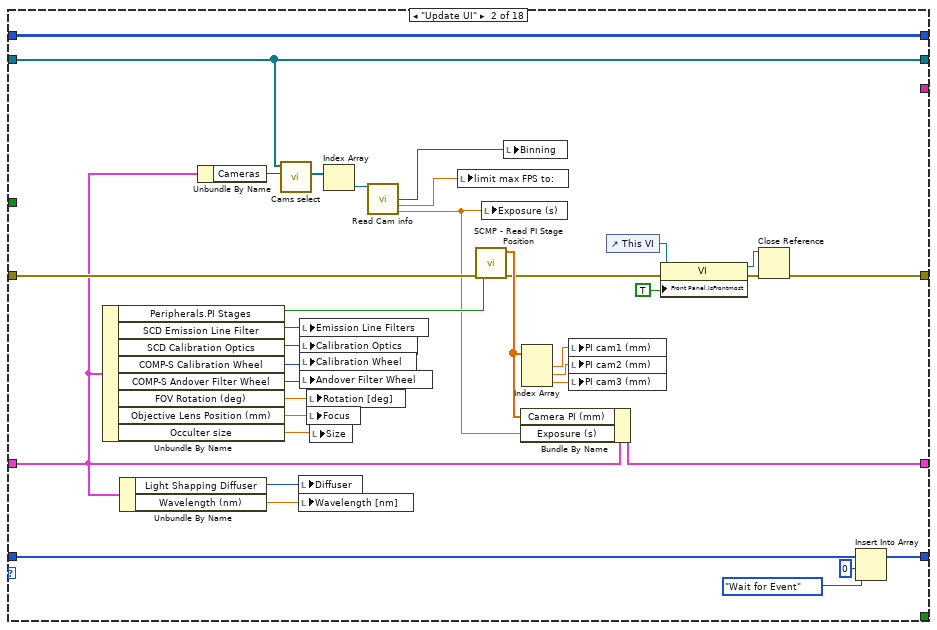
[diagram p12: hidden frame]
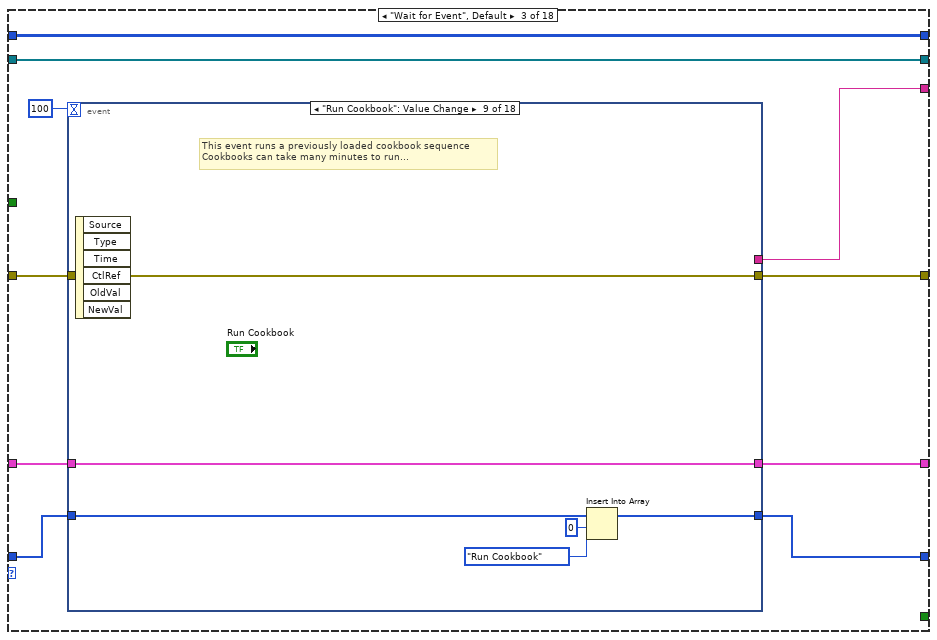
[diagram p13: hidden frame]
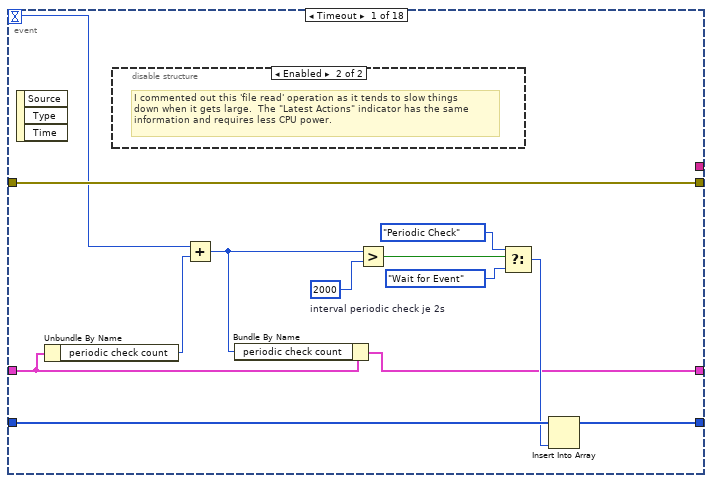
[diagram p14: hidden frame]
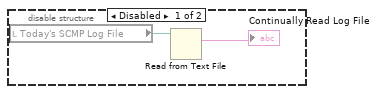
[diagram p15: hidden frame]
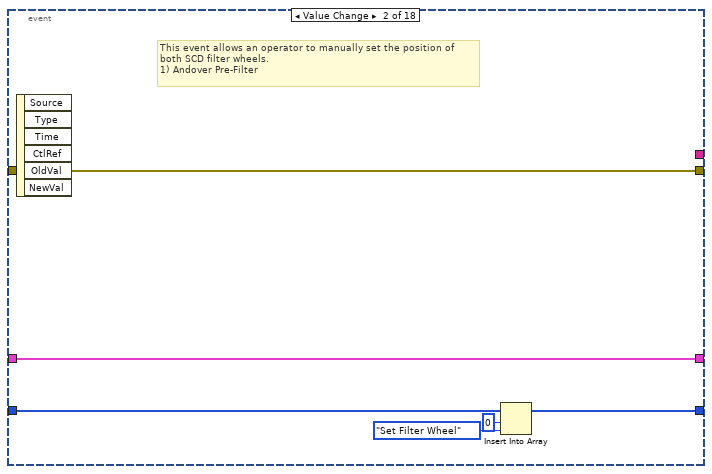
[diagram p16: hidden frame]
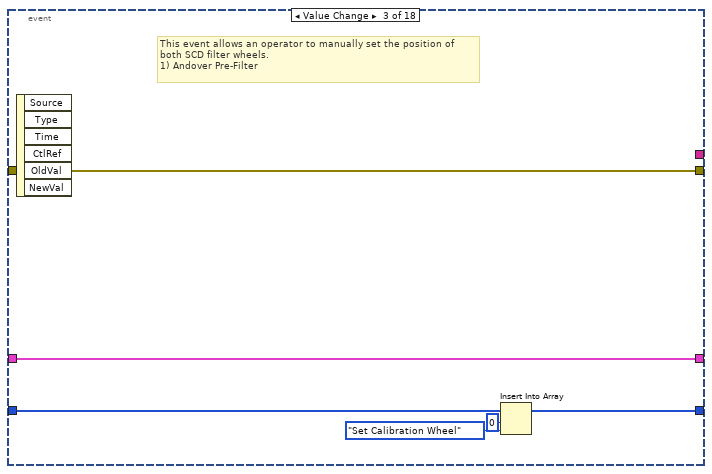
[diagram p17: hidden frame]
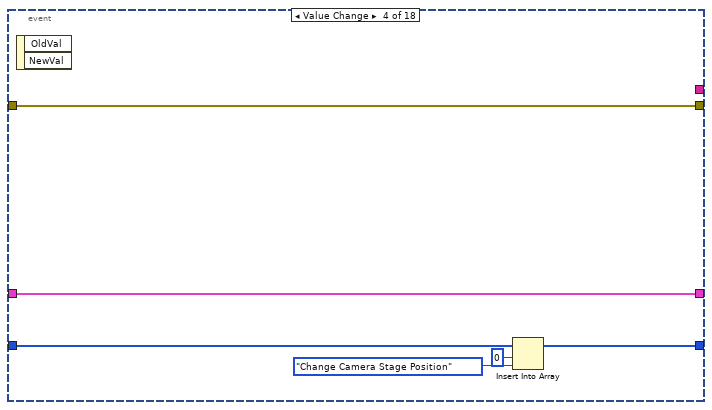
[diagram p18: hidden frame]
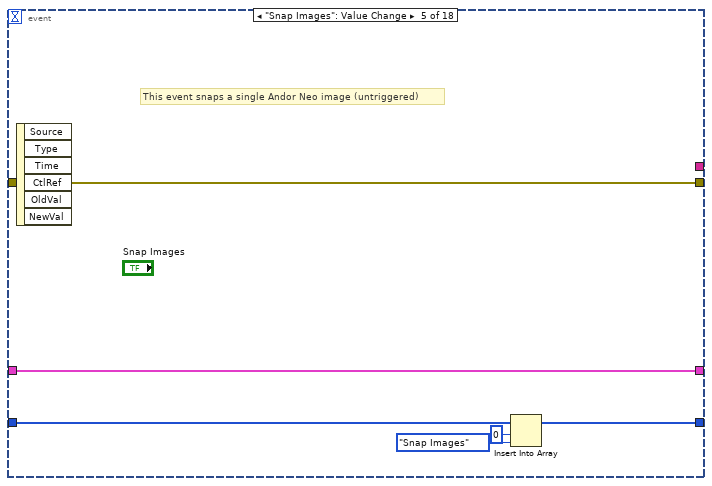
[diagram p19: hidden frame]
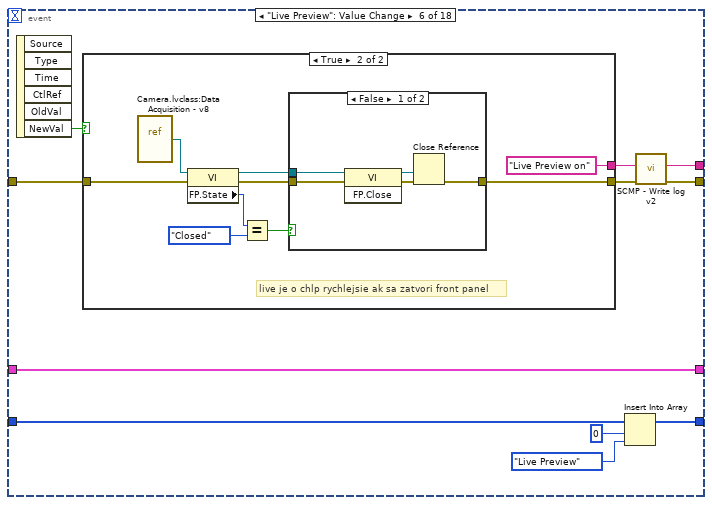
[diagram p20: hidden frame]
diagram:
  w4 = u16[][][] []  # Image Data Arr
  w14 = Main_Program_States."Initialize"  # Beginning State
  w34 = ""  # Message String Constant
  # "state queue"
  # "uz sa nepouziva"
  # "Initialization:\n1) Opens handle to camera and to Andor SDK3 DLL\n2) Starts cooling the camera to -20C and reset FPGA clock to match computer clock\n3) Sets the current camera focus stage position to -80mm.\n4) Set the Emission Line filter wheel to aperture #1 (530nm)\n5) Set the Calibration Optics filter wheel to aperture #1 (dark)"
  # "SCD uses a standard state machine architecture where each state follows from the results of a previous state.\n1) The beginning state is always \"Initialize\" which opens a connection to the Andor Neo Camera and the PI stage\n1a) A very important sub-VI in this state is the resetting of the Camera FPGA timestamp to zero at which time the computer clock is read\n2) The program then goes into a \"Wait for Event\" state which is essentially an event handler which responds to front panel user input"
  n1 = flat-sequence {
    tunnel: [w55] -> w16
    tunnel: [w54] -> w10
    tunnel: [w41] -> w15
    frame #0 {
      n2 = disable-structure "Conditional Disable Structure" shown="SCMP==COMP, Default" {
        disable-tunnel: [TRUE ("Visible") FALSE ("Visible")] -> w59
        disable-tunnel: ["    SCD" ("String") "COMP-S" ("String")] -> w54
        disable-tunnel: [u32 16711680 u32 255] -> w62
        disable-tunnel: [u32 16769505 u32 13558015] -> w61
        disable-tunnel: [T20."Disabled and Grayed Out" ("Disabled") T20."Enabled" ("Disabled")] -> w57
        disable-tunnel: [FALSE ("Visible") TRUE ("Visible")] -> w56
        disable-tunnel: [enum16{"COMP", "SCD"}."SCD" ("SCMP") enum16{"COMP", "SCD"}."COMP" ("SCMP")] -> w58
        frame condition #0 {
        }
        frame condition #1 (active) {
        }
      }
      n3 = control-ref of="This VI"() -> (w38:refnum<vi>)
      n4 = property on="Size" class="DigNum (strict)"("DisabledEnum"=w57) -> (error out=w53:errorcluster)  [unwired: 2 in, 1 out]
      n5 = global write "Globals.vi" "SCMP"(w58) -> ()
      n6 = disable-structure shown="demo==on" {
        disable-tunnel: [w66 u32 14408667] -> w55
        disable-tunnel: w61 -> [w66 _]
        disable-tunnel: [FALSE ("demo") TRUE ("demo")] -> w60
        frame condition #0 (active) {
        }
        frame condition #1 {
        }
      }
      n7 = invoke class="VI" method="Default Vals.Reinit All"(reference=w38) -> (reference out=w36:refnum<vi>, error out=w37:errorcluster)  [unwired: 2 in, 1 out]
      n8 = property on="Motors" class="Bool (strict)"(error in=w53, "DisabledEnum"=w57) -> (error out=w52:errorcluster)  [unwired: 1 in, 1 out]
      n9 = property on="Instrument" class="Str"("Text.FontSize"=u32 80 ("Text.Font:Color"), "Text.FontColor"=w62, "Text.FontBold"=TRUE ("Text.Font:Bold")) -> (error out=w40:errorcluster)  [unwired: 2 in, 1 out]
      n10 = property on="Pane" class="Pane"(error in=w52, "PaneColor"=w55) -> (error out=w39:errorcluster)  [unwired: 1 in, 1 out]
      n11 = global write "Global demo.vi" "demo"(w60) -> ()
      n12 = Close Reference(reference=w36, error in (no error)=w37) -> (error out=w35:errorcluster)
      n13 = property on="Camera Image" class="IntGraph (strict)"(error in=w35, "Visible"=w59) -> (error out=w43:errorcluster)  [unwired: 1 in, 1 out]
      n14 = property on="Camera T Image" class="IntGraph (strict)"(error in=w43, "Visible"=w56) -> (error out=w49:errorcluster)  [unwired: 1 in, 1 out]
      n15 = property on="Camera T Image Zoom" class="IntGraph (strict)"(error in=w49, "Visible"=w56) -> (error out=w48:errorcluster)  [unwired: 1 in, 1 out]
      n16 = property on="Camera R Image" class="IntGraph (strict)"(error in=w48, "Visible"=w56) -> (error out=w47:errorcluster)  [unwired: 1 in, 1 out]
      n17 = property on="Mean ADU 2" class="DigNum (strict)"(error in=w47, "Visible"=w56) -> (error out=w46:errorcluster)  [unwired: 1 in, 1 out]
      n18 = property on="Timestamp 2" class="AbsTime (strict)"(error in=w46, "Visible"=w56) -> (error out=w45:errorcluster)  [unwired: 1 in, 1 out]
      n19 = property on="Sharpness 2" class="DigNum (strict)"(error in=w45, "Visible"=w56) -> (error out=w44:errorcluster)  [unwired: 1 in, 1 out]
      n20 = property on="Histogram Graph 2" class="XYGraph (strict)"(error in=w44, "Visible"=w56) -> (error out=w50:errorcluster)  [unwired: 1 in, 1 out]
      n21 = property on="Camera FITS file path 2" class="Path"(error in=w50, "Visible"=w56) -> (error out=w51:errorcluster)  [unwired: 1 in, 1 out]
      n22 = property on="Camera 2 Temp [C}" class="WFChart (strict)"(error in=w51, "Visible"=w56) -> (error out=w42:errorcluster)  [unwired: 1 in, 1 out]
      n23 = Merge Errors(w42, w40, w39) -> (w41:errorcluster)
    }
  }
  n24 = call "SCMP - System init v2.vi"("error in (no error)"=w15, "Pane Color"=w16, "instrument"=w10) -> ("error main"=w3:errorcluster, "Cameras"=w19:refnum<class "Camera.lvclass">[], "Peripherals"=w18:T16, "cont?"=w12:bool, "Today's SCMP Engineering File"=→"Today's SCMP Eng  File":path, "Version"=→"Version":string)  [unwired: 3 in]
  n25 = Bundle By Name(cluster=T18 {"Wavelength (nm)"=530.15, "Exposure (s)"=0.05, "Tuning Delay (ms)"=200.0, "Beam Type (-1/1)"=1.0, "Tuning Voltages"=[1.111, 2.222, 3.333, 4.444], "Observer"="observer", "Light Shapping Diffuser"=enum."In Beam", "Comment"="", "Data Type"=enum."LIVE", "Mod Cycles"=1, "SCD Calibration Optics"=enum."1 - Polarizer @0, I+Q", "SCD Emission Line Filter"=enum."1-557.6nm", "Cookbook"="", "COMP-S Calibration Wheel"=enum."Dark", "COMP-S Andover Filter Wheel"=enum."530.3nm/HWB 0.34nm (Fe XIV)", "FOV Rotation (deg)"=66.0, "Objective Lens Position (mm)"=0.0, "Occulter size"=0.0, "Time End"=timestamp(3382374145.421875 s since 1904-01-01), "Acc Exposure (s)"=0.0, "Time Stamp Array"=[], "Camera Serial Number"=[], "Camera Temp"=[], "Camera PI (mm)"=[0.0, 0.0, 0.0], "Time Start"=timestamp(3382374145.421875 s since 1904-01-01), "Peripherals"={"ILX controler"=FALSE, "Zone temperatures"=FALSE, "Andor"=FALSE, "Andor 2"=FALSE, "PI Stages"=FALSE, "AISAS mechanisms"=FALSE, "AISAS Mech.lvclass"=refnum, "Zone temp ref"=variant, "FWs"=FALSE}, "FITS paths"=[], "Cameras"=enum."Andor", "load preset cbk"=FALSE, "periodic check count"=0, "COMP-S Calibration Wheel 2"=enum."Dark", "Calib"=enum."Dark", "Abso Aperture"=40.0, "Nominal Aperture"=196.0, "Pointer IP"="127.0.0.1"} ("FITS"), "Peripherals"=w18) -> (w21:T18)
  n26 = Select(t=w14, s=w12, f=Main_Program_States."Stop" ("Beginning State")) -> (s? t:f=w2:T17)
  n27 = Build Array(w2) -> (w1:T17[])
  n28 = while {
    shift-right: [w97] -> w30
    shift-left: w3 -> [w103]
    shift-right: [w98] -> _
    shift-left: w34 -> [w100]
    shift-right: [w92] -> _
    shift-left: w21 -> [w102]
    shift-right: [w93] -> w5
    shift-left: w19 -> [w101]
    shift-right: [w84] -> _
    shift-left: w1 -> [w87]
    tunnel: w12 -> [w90]
    shift-right: [w89] -> _
    shift-left: w4 -> [w88]
    stop <- w91 stop-if-true
    # "Clear Errors After\nEach Loop"
    n29 = Delete From Array(array=w87, index=0) -> (deleted portion=w86:T17, array with subset deleted=w85:T17[])  [unwired: 1 in]
    n30 = case shown="\"Run Cookbook\"" w86 {
      tunnel: w103 -> [w108 w194 w209 w392 w417 w459 w472 w525 w577 w614 w645 w677 w706 w738 w774 w792 w824 w848]
      tunnel: [w147 w175 w208 w395 w417 w453 w466 w523 w595 w612 w644 w676 w692 w735 w773 w798 w816 w849] -> w94
      tunnel: [w142 _ w204 w394 _ w452 _ w533 w572 w616 w647 w675 w708 w739 w775 w799 _ w851] -> w99
      tunnel: w102 -> [w125 w185 w207 w393 w419 w457 w470 w502 w590 w608 w640 w672 w707 w729 w769 w786 w823 w841]
      tunnel: [w141 w191 w206 w376 w419 w450 w467 w532 w579 w607 w639 w671 w691 w736 w769 w786 w823 w841] -> w92
      tunnel: w101 -> [w115 w184 w210 w383 w421 w458 w471 w505 w568 w615 w646 w685 w711 w737 w765 w793 w812 w850]
      tunnel: [w115 w184 w210 w383 w421 w456 w469 w505 w567 w615 w646 w685 w711 w737 w764 w790 w811 w850] -> w93
      tunnel: [_ _ _ _ _ _ _ _ _ _ _ _ _ _ _ _ _ TRUE ("x = y?")] -> w91
      tunnel: w90 -> [_ _ _ _ _ _ _ _ _ _ _ _ _ _ _ _ _ w838]
      tunnel: [w116 w190 w205 w384 w422 w451 w468 w519 w569 w605 w638 w669 w690 w725 w772 w796 w822 w837] -> w89
      tunnel: w88 -> [w116 w190 w205 w384 w422 _ w465 w519 w569 w605 w638 w669 w690 w725 w772 w796 w822 w837]
      tunnel: w85 -> [_ w172 w203 _ w416 w448 w464 w518 w566 w604 w637 w668 w689 w724 w758 w785 w809 _]
      tunnel: [w110 w173 w202 w379 w416 w447 w463 w517 w565 w603 w636 w667 w688 w723 w757 w784 w808 w835] -> w84
      frame "Initialize" {
        w143 = timestamp(-3600 s since 1904-01-01) ("element")
        # "Set up a grayscale color pallete for the image"
        # "scd"
        # "comp"
        n31 = control-ref of="preset cbk"() -> (w107:refnum<vi>)
        n32 = call "SCMP - Populate preset cbk ring.vi"("error in (no error)"=w108, "preset cbk ring ref"=w107) -> ("error out"=w106:errorcluster)  [unwired: 9 in]
        n33 = control-ref of="PI cam1 (mm)"() -> (w127:refnum<vi>)
        n34 = control-ref of="PI cam2 (mm)"() -> (w128:refnum<vi>)
        n35 = control-ref of="PI cam3 (mm)"() -> (w129:refnum<vi>)
        n36 = for {
          N: 256 -> [_]
          tunnel: [w151] -> w122 mode=indexing
          i -> [w152]
          n37 = Multiply(x=65793, y=w152) -> (x*y=w151:i32)
        }
        n38 = for {
          tunnel: w115 -> [w149] mode=indexing
          tunnel: [w148] -> w114 mode=indexing
          n39 = call-dynamic "Read Cam info.vi"("Camera in"=w149) -> ("SerialNumber"=w148:string)  [unwired: 5 in, 9 out]
        }
        n40 = property on="Run Cookbook" class="Bool"(error in=w106, "DisabledEnum"=T20."Disabled and Grayed Out" ("Disabled")) -> (error out=w105:errorcluster)  [unwired: 1 in, 1 out]
        n41 = Build Array(w127, w128, w129) -> (w126:refnum<vi>[])
        n42 = call "SCMP - Set PI indicators.vi"("PI refs"=w126, "error in (no error)"=w105, "FITS Header in"=w125) -> ("error out"=w121:errorcluster, "FITS Header out"=w124:T18)  [unwired: 7 in]
        n43 = property on="Camera T Image" class="IntGraph (strict)"(error in=w121, "Color Table"=w122, "ZScale.UniformMarker"=TRUE ("Z Scale.Uniform Marker Spacing?")) -> (error out=w120:errorcluster)  [unwired: 1 in, 1 out]
        n44 = local read "Selected Cookbook"() -> (w146:path)
        n45 = control-ref of="Emission Line Filters"() -> (w133:refnum<vi>)
        n46 = control-ref of="Calibration Optics"() -> (w132:refnum<vi>)
        n47 = control-ref of="Andover Filter Wheel"() -> (w135:refnum<vi>)
        n48 = control-ref of="Calibration Wheel"() -> (w134:refnum<vi>)
        n49 = Build Array(w143, w143, w143, w143) -> (w118:timestamp[])
        n50 = Build Array(w135, w134, w133, w132) -> (w131:refnum<vi>[])
        n51 = Strip Path(path=w146) -> (name=w145:string)  [unwired: 1 out]
        n52 = Initialize Array(path "", 4 ("dimension size")) -> (w111:path[])
        n53 = call "SCMP - FW init.vi"("FW refs"=w131, "error in (no error)"=w120, "FITS Header in"=w124) -> ("error out"=w144:errorcluster, "FITS Header out"=w139:T18)  [unwired: 7 in]
        n54 = call "SCMP Rotation and Focus Check.vi"("error in"=w144, "FITS Header In"=w139) -> ("error out"=w140:errorcluster, "FITS Header Out"=w138:T18)  [unwired: 5 in, 3 out]
        n55 = call "Init Load.vi"("error in (no error)"=w140, "FITS Header in"=w138) -> ("error out"=w130:errorcluster, "Motors (off/on)"=w136:bool, "FITS Header out"=w137:T18)  [unwired: 7 in]
        n56 = Bundle By Name(cluster=w137, "Cookbook"=w145, "Time Stamp Array"=w118, "Cameras"=Cameras_select."Andor", "Camera Serial Number"=w114, "FITS paths"=w111) -> (w141:T18)
        n57 = local write "Motors"(w136) -> ()
        n58 = case shown="No Error" w130 {
          selector: w130 -> [w156 w166]
          tunnel: [w154 w163] -> w142
          tunnel: [w155 w165] -> w147
          tunnel: [Main_Program_States."Update UI" ("Beginning State") w159] -> w109
          frame No Error {
            n59 = call "SCMP - Write log v2.vi"("Error to log"=w156, "data"="Program Started") -> ("error out"=w155:errorcluster, "Last Log Entry"=w154:string, "Today's SCMP Log File"=→"Today's SCMP Log File":path)  [unwired: 7 in]
          }
          frame Error {
            n60 = global read "Global demo.vi" "demo"() -> (w160:bool)
            n61 = call "SCMP - Write log v2.vi"("Error to log"=w166, "data"="FW Init Failure!") -> ("error out"=w165:errorcluster, "Last Log Entry"=w163:string)  [unwired: 7 in, 1 out]
            n62 = Select(t=Main_Program_States."Update UI" ("Beginning State"), s=w160, f=Main_Program_States."Stop" ("Beginning State")) -> (s? t:f=w159:T17)
          }
        }
        n63 = Build Array(w109) -> (w110:T17[])
      }
      frame "Update UI" {
        n64 = Unbundle By Name(w185) -> ("Peripherals.PI Stages"=w193:bool, "SCD Emission Line Filter"=w195:T9, "SCD Calibration Optics"=w196:T4, "COMP-S Calibration Wheel"=w197:T7, "COMP-S Andover Filter Wheel"=w198:T6, "FOV Rotation (deg)"=w171:dbl, "Objective Lens Position (mm)"=w170:T5, "Occulter size"=w169:dbl)
        n65 = Unbundle By Name(w185) -> ("Light Shapping Diffuser"=w189:T10, "Wavelength (nm)"=w167:dbl)
        n66 = Unbundle By Name(w185) -> ("Cameras"=w188:T12)
        n67 = call "Cams select.vi"("Cameras"=w188, "Cameras in"=w184) -> ("Cams selection"=w187:refnum<class "Camera.lvclass">[])  [unwired: 8 in, 1 out]
        n68 = local write "Diffuser"(w189) -> ()
        n69 = local write "Wavelength [nm]"(w167) -> ()
        n70 = local write "Emission Line Filters"(w195) -> ()
        n71 = local write "Calibration Optics"(w196) -> ()
        n72 = local write "Calibration Wheel"(w197) -> ()
        n73 = local write "Andover Filter Wheel"(w198) -> ()
        n74 = local write "Rotation [deg]"(w171) -> ()
        n75 = local write "Focus"(w170) -> ()
        n76 = local write "Size"(w169) -> ()
        n77 = Index Array(array=w187) -> (element=w186:refnum<class "Camera.lvclass">)  [unwired: 1 in]
        n78 = call-dynamic "Read Cam info.vi"("Camera in"=w186) -> ("Binning"=w181:T8, "FPS"=w182:dbl, "Exposure [s]"=w183:dbl)  [unwired: 5 in, 7 out]
        n79 = local write "limit max FPS to:"(w182) -> ()
        n80 = call "SCMP - Read PI Stage Position.vi"("Enable"=w193, "error in (no error)"=w194) -> ("error out"=w176:errorcluster, "Output Array"=w192:dbl[])  [unwired: 8 in]
        n81 = local write "Exposure (s)"(w183) -> ()
        n82 = local write "Binning"(w181) -> ()
        n83 = Bundle By Name(cluster=w185, "Camera PI (mm)"=w192, "Exposure (s)"=w183) -> (w191:T18)
        n84 = Index Array(array=w192) -> (element #1=w199:dbl, element #2=w200:dbl, element #3=w201:dbl)  [unwired: 3 in]
        n85 = local write "PI cam1 (mm)"(w199) -> ()
        n86 = local write "PI cam2 (mm)"(w200) -> ()
        n87 = local write "PI cam3 (mm)"(w201) -> ()
        n88 = control-ref of="This VI"() -> (w177:refnum<vi>)
        n89 = property class="VI"(reference=w177, error in=w176, "Front Panel.IsFrontmost"=TRUE ("Front Panel Window:Is Frontmost")) -> (reference out=w180:refnum<vi>, error out=w179:errorcluster)
        n90 = Close Reference(reference=w180, error in (no error)=w179) -> (error out=w175:errorcluster)
        n91 = Insert Into Array(array=w172, index=0, new element=Main_Program_States."Wait for Event" ("Next State")) -> (w173:T17[])
      }
      frame "Wait for Event", Default {
        n92 = event shown="[8] \"Run Cookbook\": Value Change" {
          selector: _ -> [_ _ _ _ _ _ _ _ _ _ _ _ _ _ _ _ _ _]
          dyn-events: _ -> [_ _ _ _ _ _ _ _ _ _ _ _ _ _ _ _ _ _]
          timeout: 100 -> [w220 _ _ _ _ _ _ _ _ _ _ _ _ _ _ _ _ _]
          tunnel: w209 -> [w224 w232 w238 w244 w250 w254 w286 w294 w300 w306 w312 w325 w338 w351 w357 w363 w369 w375]
          tunnel: [w224 w232 w238 w244 w250 w260 w286 w294 w300 w306 w312 w323 w336 w349 w357 w363 w369 w375] -> w208
          tunnel: w207 -> [w214 w231 w237 w243 w249 w261 w285 w289 w299 w305 w311 w322 w335 w348 w356 w362 w368 w374]
          tunnel: [w212 w231 w237 w243 w249 w261 w285 w287 w299 w305 w311 w320 w333 w346 w356 w362 w368 w374] -> w206
          tunnel: [_ _ _ _ _ w259 _ _ _ _ _ _ _ _ _ _ _ _] -> w204
          tunnel: w203 -> [w223 w230 w236 w242 w248 w258 w284 w293 w298 w304 w310 w316 w329 w342 w355 w361 w367 w373]
          tunnel: [w222 w229 w235 w241 w247 w257 w283 w292 w297 w303 w309 w315 w328 w341 w354 w360 w366 w372] -> w202
          event Timeout {
            w219 = 2000  # interval periodic check je 2s
            n93 = event-data() -> ()  [unwired: 1 in, 3 out]
            n94 = Unbundle By Name(w214) -> ("periodic check count"=w221:i32)
            n95 = disable-structure shown="Enabled" {
              frame Disabled {
                n96 = local read "Today's SCMP Log File"() -> (w226:path)
                n97 = Read from Text File(file (use dialog)=w226) -> (text=→"Continually Read Log File":string)  [unwired: 3 in, 3 out]
              }
              frame Enabled {
                # "I commented out this 'file read' operation as it tends to slow things\ndown when it gets large.  The \"Latest Actions\" indicator has the same\ninformation and requires less CPU power."
              }
            }
            n98 = Add(x=w220, y=w221) -> (x+y=w213:i32)
            n99 = Bundle By Name(cluster=w214, "periodic check count"=w213) -> (w212:T18)
            n100 = Greater?(x=w213, y=w219) -> (0:w217:bool)
            n101 = Select(t=Main_Program_States."Periodic Check" ("Next State"), s=w217, f=Main_Program_States."Wait for Event") -> (s? t:f=w215:T17)
            n102 = Insert Into Array(array=w223, new element=w215) -> (w222:T17[])  [unwired: 1 in]
          }
          event Value Change {
            # "This event allows an operator to manually set the position of\nboth SCD filter wheels.  \n1) Andover Pre-Filter"
            n103 = event-data() -> ()  [unwired: 1 in, 6 out]
            n104 = Insert Into Array(array=w230, index=0, new element=Main_Program_States."Set Filter Wheel" ("Next State")) -> (w229:T17[])
          }
          event Value Change {
            # "This event allows an operator to manually set the position of\nboth SCD filter wheels.  \n1) Andover Pre-Filter"
            n105 = event-data() -> ()  [unwired: 1 in, 6 out]
            n106 = Insert Into Array(array=w236, index=0, new element=Main_Program_States."Set Calibration Wheel" ("Next State")) -> (w235:T17[])
          }
          event Value Change {
            n107 = event-data() -> ()  [unwired: 1 in, 2 out]
            n108 = Insert Into Array(array=w242, index=0, new element=Main_Program_States."Change Camera Stage Position" ("Next State")) -> (w241:T17[])
          }
          event "Snap Images": Value Change {
            # "This event snaps a single Andor Neo image (untriggered)"
            n109 = event-data() -> ()  [unwired: 1 in, 6 out]
            n110 = Insert Into Array(array=w248, index=0, new element=Main_Program_States."Snap Images" ("Next State")) -> (w247:T17[])
          }
          event "Live Preview": Value Change {
            n111 = event-data() -> ("NewVal"=w252:bool)  [unwired: 1 in, 5 out]
            n112 = case shown="True" w252 {
              tunnel: w254 -> [w263 w269]
              tunnel: [w263 w272] -> w253
              tunnel: ["Live Preview off" ("Last Log Entry") "Live Preview on" ("Last Log Entry")] -> w251
              frame False {
              }
              frame True {
                # "live je o chlp rychlejsie ak sa zatvori front panel"
                n113 = vi-ref "Camera.lvclass:Data Acquisition - v8.vi"() -> (w270:refnum<vi>)
                n114 = property class="VI"(reference=w270, error in=w269) -> (reference out=w264:refnum<vi>, error out=w265:errorcluster, "FP.State"=w268:T21)
                n115 = Equal?(x=w268, y=T21."Closed") -> (x = y?=w266:bool)
                n116 = case shown="False" w266 {
                  tunnel: [w275 w280] -> w272
                  tunnel: w265 -> [w274 w279]
                  tunnel: w264 -> [w273 w278]
                  frame False {
                    n117 = invoke class="VI" method="FP.Close"(reference=w273, error in=w274) -> (reference out=w276:refnum<vi>, error out=w277:errorcluster)  [unwired: 1 in, 1 out]
                    n118 = Close Reference(reference=w276, error in (no error)=w277) -> (error out=w275:errorcluster)
                  }
                  frame True {
                    n119 = Close Reference(reference=w278, error in (no error)=w279) -> (error out=w280:errorcluster)
                  }
                }
              }
            }
            n120 = Insert Into Array(array=w258, index=0, new element=Main_Program_States."Live Preview" ("Next State")) -> (w257:T17[])
            n121 = call "SCMP - Write log v2.vi"("Error to log"=w253, "data"=w251) -> ("error out"=w260:errorcluster, "Last Log Entry"=w259:string)  [unwired: 7 in, 1 out]
          }
          event "Load Cookbook": Value Change {
            # "This event lets an observer select a cookbook to 'run'"
            n122 = event-data() -> ()  [unwired: 1 in, 6 out]
            n123 = Insert Into Array(array=w284, index=0, new element=Main_Program_States."Load Cookbook" ("Next State")) -> (w283:T17[])
          }
          event "preset cbk": Value Change {
            # "This event load preset cookbook"
            n124 = event-data() -> ()  [unwired: 1 in, 6 out]
            n125 = Bundle By Name(cluster=w289, "load preset cbk"=TRUE) -> (w287:T18)
            n126 = Insert Into Array(array=w293, index=0, new element=Main_Program_States."Load Cookbook" ("Next State")) -> (w292:T17[])
          }
          event "Run Cookbook": Value Change {
            # "This event runs a previously loaded cookbook sequence\nCookbooks can take many minutes to run..."
            n127 = event-data() -> ()  [unwired: 1 in, 6 out]
            n128 = Insert Into Array(array=w298, index=0, new element=Main_Program_States."Run Cookbook" ("Next State")) -> (w297:T17[])
          }
          event "Move AISAS Mechanisms": Value Change {
            n129 = event-data() -> ()  [unwired: 1 in, 2 out]
            n130 = Insert Into Array(array=w304, index=0, new element=Main_Program_States."Move AISAS Mechanisms" ("Next State")) -> (w303:T17[])
          }
          event "Motors": Value Change {
            n131 = event-data() -> ()  [unwired: 1 in, 2 out]
            n132 = Insert Into Array(array=w310, index=0, new element=Main_Program_States."AISAS Motors on/off" ("Next State")) -> (w309:T17[])
          }
          event Value Change {
            n133 = event-data() -> ()  [unwired: 1 in, 6 out]
            n134 = Unbundle By Name(w322) -> ("Peripherals.AISAS Mech.lvclass"=w324:refnum<class "AISAS Mech.lvclass">)
            n135 = To Variant(anything="Diffuser") -> (Variant=w319:variant)
            n136 = call "Write Move Motor.vi"("error in (no error)"=w325, "Desired Value"=w319, "Motor"=motor."Diffuser ", "AISAS Mech in"=w324) -> ("error out"=w323:errorcluster, "AISAS Mech out"=w321:refnum<class "AISAS Mech.lvclass">)  [unwired: 6 in]
            n137 = Bundle By Name(cluster=w322, "Peripherals.AISAS Mech.lvclass"=w321) -> (w320:T18)
            n138 = Insert Into Array(array=w316, index=0, new element=Main_Program_States."AISAS Move" ("Next State")) -> (w315:T17[])
          }
          event Value Change {
            n139 = event-data() -> ()  [unwired: 1 in, 6 out]
            n140 = Unbundle By Name(w335) -> ("Peripherals.AISAS Mech.lvclass"=w337:refnum<class "AISAS Mech.lvclass">)
            n141 = To Variant(anything="Rotation [deg]") -> (Variant=w332:variant)
            n142 = call "Write Move Motor.vi"("error in (no error)"=w338, "Desired Value"=w332, "Motor"=motor."Rotation", "AISAS Mech in"=w337) -> ("error out"=w336:errorcluster, "AISAS Mech out"=w334:refnum<class "AISAS Mech.lvclass">)  [unwired: 6 in]
            n143 = Bundle By Name(cluster=w335, "Peripherals.AISAS Mech.lvclass"=w334) -> (w333:T18)
            n144 = Insert Into Array(array=w329, index=0, new element=Main_Program_States."AISAS Move" ("Next State")) -> (w328:T17[])
          }
          event Value Change {
            n145 = event-data() -> ()  [unwired: 1 in, 6 out]
            n146 = Unbundle By Name(w348) -> ("Peripherals.AISAS Mech.lvclass"=w350:refnum<class "AISAS Mech.lvclass">)
            n147 = To Variant(anything="Focus") -> (Variant=w345:variant)
            n148 = call "Write Move Motor.vi"("error in (no error)"=w351, "Desired Value"=w345, "Motor"=motor."Focus", "AISAS Mech in"=w350) -> ("error out"=w349:errorcluster, "AISAS Mech out"=w347:refnum<class "AISAS Mech.lvclass">)  [unwired: 6 in]
            n149 = Bundle By Name(cluster=w348, "Peripherals.AISAS Mech.lvclass"=w347) -> (w346:T18)
            n150 = Insert Into Array(array=w342, index=0, new element=Main_Program_States."AISAS Move" ("Next State")) -> (w341:T17[])
          }
          event "Exposure (s)": Value Change {
            n151 = event-data() -> ()  [unwired: 1 in, 2 out]
            n152 = Insert Into Array(array=w355, index=0, new element=Main_Program_States."Change Camera Exposure" ("Next State")) -> (w354:T17[])
          }
          event Value Change {
            n153 = event-data() -> ()  [unwired: 1 in, 3 out]
            n154 = Insert Into Array(array=w361, index=0, new element=Main_Program_States."Set Camera AOI" ("Next State")) -> (w360:T17[])
          }
          event "Andor Adv Settings": Value Change {
            n155 = event-data() -> ()  [unwired: 1 in, 2 out]
            n156 = Insert Into Array(array=w367, index=0, new element=Main_Program_States."Andor Adv Settings" ("Next State")) -> (w366:T17[])
          }
          event "Stop": Value Change {
            # "This event causes the SCD program to terminate"
            n157 = event-data() -> ()  [unwired: 1 in, 1 out]
            n158 = Insert Into Array(array=w373, index=0, new element=Main_Program_States."Stop" ("Next State")) -> (w372:T17[])
          }
        }
      }
      frame "Periodic Check" {
        w379 = T17[] [enum."Wait for Event"] items=["Initialize", "Wait for Event", "Periodic Check", "Update UI", "Update Camera UI", "Load Cookbook", "Run Cookbook", "Snap Images", "Live Preview", "Set Filter Wheel", "Set Calibration Wheel", "AISAS Motors on/off", "AISAS Move", "Move AISAS Mechanisms", "Stop", "Change Camera Exposure", "Change Camera Stage Position", "Set Camera AOI", "Andor Adv Settings", "Update Image", "Run Dark", "Calib acq", "Process Calib"]
        # "funkcia AISAS auto off:\nvypnutie tlac. Motors v pripade chyby"
        # "2sec interval (po event timeout case)"
        n159 = for {
          tunnel: [w403] -> w382 mode=indexing
          tunnel: w392 -> [w401]
          tunnel: [w402] -> w397
          tunnel: w383 -> [w400] mode=indexing
          n160 = call-dynamic "Cam temp.vi"("error in (no error)"=w401, "Camera.lvclass"=w400) -> ("error out"=w402:errorcluster, "Temp"=w403:dbl)  [unwired: 8 in]
        }
        n161 = Index Array(array=w382) -> (element #1=→"Camera 1 Temp [C}":dbl, element #2=→"Camera 2 Temp [C}":dbl)  [unwired: 2 in]
        n162 = Bundle By Name(cluster=w393, "Observer"="Observer", "Comment"="Comment", "Camera Temp"=w382, "Occulter size"="Size") -> (w390:T18)
        n163 = Unbundle By Name(w390) -> ("Peripherals"=w391:T16)
        n164 = call "Check.vi"("Peripherals in"=w391, "error in (no error)"=w397) -> ("error out"=w387:errorcluster, "auto off?"=w385:bool, "Peripherals out"=w389:T16, "auto off resp"=w396:string)  [unwired: 5 in, 1 out]
        n165 = Bundle By Name(cluster=w390, "Peripherals"=w389) -> (w378:T18)
        n166 = case shown="True" w385 {
          tunnel: w387 -> [w404 w405]
          tunnel: [w404 w407] -> w386
          frame False {
          }
          frame True {
            n167 = property on="Motors" class="Bool (strict)"("Val(Sgnl)"=FALSE ("Value (Signaling)")) -> (error out=w406:errorcluster)  [unwired: 2 in, 1 out]
            n168 = Merge Errors(w405, w406) -> (w407:errorcluster)
          }
        }
        n169 = case shown="Error" w386 {
          selector: w386 -> [w410 w411]
          tunnel: [w410 w415] -> w395
          tunnel: w396 -> [_ w412]
          tunnel: ["" ("Last Log Entry") w414] -> w394
          frame No Error {
          }
          frame Error {
            n170 = call "SCMP - Write log v2.vi"("Error to log"=w411, "data to end"=w412, "data"="AISAS Check ") -> ("error out"=w415:errorcluster, "Last Log Entry"=w414:string)  [unwired: 6 in, 1 out]
          }
        }
        n171 = Bundle By Name(cluster=w378, "periodic check count"=0) -> (w376:T18)
      }
      frame "Update Image" {
        n172 = Unbundle By Name(w419) -> ("FITS paths"=w420:path[])
        n173 = Index Array(array=w422) -> (element #1=w424:u32[][], element #2=w423:u32[][])  [unwired: 6 in]
        n174 = Index Array(array=w420) -> (element #1=→"Camera FITS file path":path, element #2=→"Camera FITS file path 2":path)  [unwired: 2 in]
        n175 = call "SCD - Determine Image Sharpness from 2D Derivative.vi"("Image In"=w424) -> ("Sharpness"=→"Sharpness":dbl)  [unwired: 9 in, 1 out]
        n176 = call "Neo - Calculate Image Statistics and Histogram2.vi"("Image In"=w424) -> ("Histogram Graph"=→"Histogram Graph":T2, "Mean ADU"=→"Mean ADU":dbl)  [unwired: 8 in, 1 out]
        n177 = call "Neo - Calculate Image Statistics and Histogram2.vi"("Image In"=w423) -> ("Histogram Graph"=→"Histogram Graph 2":T2, "Mean ADU"=→"Mean ADU 2":dbl)  [unwired: 8 in, 1 out]
        n178 = call "SCD - Determine Image Sharpness from 2D Derivative.vi"("Image In"=w423) -> ("Sharpness"=→"Sharpness 2":dbl)  [unwired: 9 in, 1 out]
        n179 = Array Size(array=w424) -> (size(s)=w426:i32[])
        n180 = Index Array(array=w426) -> (element=w425:i32)  [unwired: 1 in]
        n181 = disable-structure shown="SCMP==COMP, Default" {
          disable-tunnel: w424 -> [w442 w443]
          disable-tunnel: w423 -> [w441 _]
          disable-tunnel: w425 -> [w437 _]
          frame condition #0 (active) {
            n182 = property on="Camera R Image" class="IntGraph (strict)"("YScale.Maximum"=w437) -> (error out=w438:errorcluster)  [unwired: 2 in, 1 out]
            n183 = Divide(x=w437, y=2) -> (x/y=w439:dbl)
            n184 = property on="Camera T Image Zoom" class="IntGraph (strict)"("YScale.Maximum"=w439) -> ()  [unwired: 2 in, 2 out]
            n185 = property on="Camera T Image" class="IntGraph (strict)"(error in=w438, "YScale.Maximum"=w437) -> ()  [unwired: 1 in, 2 out]
            "Camera T Image Zoom" <- w442
            "Camera R Image" <- w441
            "Camera T Image" <- w442
          }
          frame condition #1 {
            "Camera Image" <- w443
          }
        }
        n186 = Unbundle By Name(w419) -> ("Time Stamp Array"=w418:timestamp[])
        n187 = Index Array(array=w418) -> (element #1=→"Timestamp":timestamp, element #2=→"Timestamp 2":timestamp)  [unwired: 2 in]
      }
      frame "Snap Images" {
        n188 = call "Snap.vi"("Save Data to FITS? (F)"="Save Data to FITS?", "error in"=w459, "FITS/UI"=w457, "Cameras in"=w458) -> ("error out"=w454:errorcluster, "FITS/UI out"=w450:T18, "Image Data Arr"=w451:u16[][][], "Cameras out"=w456:refnum<class "Camera.lvclass">[])  [unwired: 4 in]
        n189 = call "SCMP - Write log v2.vi"("Error to log"=w454, "data"="Snap Single Image") -> ("error out"=w453:errorcluster, "Last Log Entry"=w452:string)  [unwired: 7 in, 1 out]
        n190 = Insert Into Array(array=w448, index=0, new element #1=Main_Program_States."Update Image" ("Next State"), new element #2=Main_Program_States."Wait for Event" ("new element/subarray")) -> (w447:T17[])
      }
      frame "Live Preview" {
        n191 = case shown="True" "Live Preview" {
          tunnel: w472 -> [w476 w495]
          tunnel: w471 -> [w474 w480]
          tunnel: w470 -> [w475 w493]
          tunnel: [w474 w479] -> w469
          tunnel: [w476 w494] -> w466
          tunnel: [w477 w484] -> w468
          tunnel: [w475 w487] -> w467
          tunnel: w465 -> [w477 _]
          tunnel: [w473 w478] -> w462
          frame False {
            w473 = T17[] [enum."Wait for Event"] items=["Initialize", "Wait for Event", "Periodic Check", "Update UI", "Update Camera UI", "Load Cookbook", "Run Cookbook", "Snap Images", "Live Preview", "Set Filter Wheel", "Set Calibration Wheel", "AISAS Motors on/off", "AISAS Move", "Move AISAS Mechanisms", "Stop", "Change Camera Exposure", "Change Camera Stage Position", "Set Camera AOI", "Andor Adv Settings", "Update Image", "Run Dark", "Calib acq", "Process Calib"]
          }
          frame True {
            w478 = T17[] [enum."Update Image", enum."Wait for Event", enum."Live Preview"] items=["Initialize", "Wait for Event", "Periodic Check", "Update UI", "Update Camera UI", "Load Cookbook", "Run Cookbook", "Snap Images", "Live Preview", "Set Filter Wheel", "Set Calibration Wheel", "AISAS Motors on/off", "AISAS Move", "Move AISAS Mechanisms", "Stop", "Change Camera Exposure", "Change Camera Stage Position", "Set Camera AOI", "Andor Adv Settings", "Update Image", "Run Dark", "Calib acq", "Process Calib"]
            n192 = disable-structure shown="SCMP==COMP, Default" {
              disable-tunnel: "Wavelength [nm]" -> [w497 w498]
              disable-tunnel: [w496 w499] -> w489
              frame condition #0 (active) {
                n193 = call "CoMP-S Tune LCVR.vi"("Wavelength (nm)"=w497) -> ("Required LCVR Voltages"=w496:dbl[])  [unwired: 9 in, 1 out]
              }
              frame condition #1 {
                n194 = call "SCD - Use Global Variables to Compute LCVR Voltages.vi"("Wavelength (nm)"=w498) -> ("Required LCVR Voltages"=w499:dbl[])  [unwired: 1 in, 1 out]
              }
            }
            n195 = Bundle By Name(cluster=w493, "Tuning Voltages"=w489, "Wavelength (nm)"="Wavelength [nm]") -> (w490:T18)
            n196 = local read "Save Data to FITS?"() -> (w483:bool)
            n197 = Build Array(w489) -> (w488:dbl[][])
            n198 = Build Array(w490) -> (w491:T18[])
            n199 = call "Data Acquisition - v8.vi"("Cameras in"=w480, "Save to FITS?"=w483, "error in"=w495, "LCVR Voltages"=w488, "Headers In"=w491) -> ("Cameras out"=w479:refnum<class "Camera.lvclass">[], "Image data"=w486:u32[][], "Image data2"=w485:u32[][], "Headers Out"=w482:T18[], "error out"=w494:errorcluster)  [unwired: 5 in, 1 out]
            n200 = Index Array(array=w482, index=0) -> (element=w487:T18)
            n201 = Build Array(w486, w485) -> (w484:u32[][][])
          }
        }
        n202 = Insert Into Array(array=w464, index=0, new element=w462) -> (w463:T17[])
      }
      frame "Load Cookbook" {
        n203 = Unbundle By Name(w502) -> ("load preset cbk"=w510:bool)
        n204 = Unbundle By Name(w502) -> ("Cameras"=w501:T12)
        n205 = control-ref of="preset cbk"() -> (w500:refnum<vi>)
        n206 = call "SCMP - Read Cookbook.vi"("error in"=w525, "load preset cbk?"=w510, "preset cbk ring ref"=w500) -> ("error out"=w507:errorcluster, "Recipe Files"=→"Recipe Files":string[], "# of Recipes"=w527:i16, "Cookbook"=→"Cookbook":T13, "min Cookbook Exposure [s]"=w521:dbl, "Selected Cookbook"=w522:path, "Cookbook Comments"=→"Cookbook Comments":string)  [unwired: 2 in]
        "Selected Cookbook" <- w522
        "min Cookbook Exposure [s]" <- w521
        n207 = call "Cams select.vi"("Cameras"=w501, "Cameras in"=w505) -> ("Cams selection"=w504:refnum<class "Camera.lvclass">[])  [unwired: 8 in, 1 out]
        n208 = Index Array(array=w504) -> (element=w503:refnum<class "Camera.lvclass">)  [unwired: 1 in]
        n209 = Greater Than 0?(x=w521) -> (x > 0?=w520:bool)
        n210 = case shown="True" w520 {
          tunnel: w521 -> [_ w538]
          tunnel: w507 -> [w535 w541]
          tunnel: [w535 w540] -> w506
          tunnel: w503 -> [_ w539]
          frame False {
          }
          frame True {
            n211 = call-dynamic "Check FPS.vi"("Set Exp or Check Fps (Set Exp)"=enum16{"Set Exp", "Check FPS"}."Check FPS", "error in (no error)"=w541, "Exposure [s]"=w538, "Camera in"=w539) -> ("error out"=w540:errorcluster, "FPS"=w536:dbl)  [unwired: 5 in, 1 out]
            n212 = local write "limit max FPS to:"(w536) -> ()
          }
        }
        n213 = Unbundle By Name(w506) -> ("status"=w511:bool)
        n214 = case shown="No Error" w506 {
          selector: w506 -> [w544 w553]
          tunnel: w527 -> [w550 _]
          tunnel: w522 -> [w548 w557]
          tunnel: [w549 w555] -> w534
          tunnel: [w543 w552] -> w530
          frame No Error {
            n215 = Strip Path(path=w548) -> (name=w546:string)  [unwired: 1 out]
            "cbk name" <- w546
            n216 = property on="Run Cookbook" class="Bool"(error in=w544, "DisabledEnum"=T20."Enabled" ("Disabled")) -> (error out=w543:errorcluster)  [unwired: 1 in, 1 out]
            n217 = Concatenate Strings("Loaded Cookbook" ("data"), "\t", w546) -> (w549:string)
            "# of Recipes" <- w550
          }
          frame Error {
            n218 = Strip Path(path=w557) -> (name=w556:string)  [unwired: 1 out]
            n219 = property on="Run Cookbook" class="Bool"(error in=w553, "DisabledEnum"=T20."Disabled and Grayed Out" ("Disabled")) -> (error out=w552:errorcluster)  [unwired: 1 in, 1 out]
            n220 = Concatenate Strings("Error Loading Cookbook" ("data"), "\t", w556) -> (w555:string)
          }
        }
        n221 = Not(x=w511) -> (.not. x?=w508:bool)
        n222 = And(x=w508, y=w510) -> (x .and. y?=w509:bool)
        n223 = Strip Path(path=w522) -> (name=w531:string)  [unwired: 1 out]
        n224 = Select(t=Main_Program_States."Run Cookbook", s=w509, f=Main_Program_States."Wait for Event" ("Next State")) -> (s? t:f=w512:T17)
        n225 = Bundle By Name(cluster=w502, "Cookbook"=w531, "load preset cbk"=FALSE) -> (w532:T18)
        n226 = call "SCMP - Write log v2.vi"("Error to log"=w530, "data"=w534) -> ("error out"=w524:errorcluster, "Last Log Entry"=w533:string)  [unwired: 7 in, 1 out]
        n227 = Insert Into Array(array=w518, index=0, new element=w512) -> (w517:T17[])
        n228 = call <vilib>:"Clear Errors.vi"("error in (no error)"=w524) -> ("error out"=w523:errorcluster)  [unwired: 5 in, 1 out]
      }
      frame "Run Cookbook" {
        # "beep na konci ak cbk trval dlhsie ako 60 sec"
        n229 = local read "cbk name"() -> (w573:string)
        n230 = Concatenate Strings("Run Cookbook" ("data"), "\t", w573) -> (w578:string)
        n231 = call "SCMP - Write log v2.vi"("Error to log"=w577, "data"=w578) -> ("error out"=w576:errorcluster, "Last Log Entry"=w570:string)  [unwired: 7 in, 1 out]
        n232 = flat-sequence {
          tunnel: [w600] -> w587
          tunnel: w576 -> [w600]
          tunnel: [w599] -> w584
          frame #0 {
            n233 = Get Date/Time In Seconds() -> (seconds since 1Jan1904=w599:timestamp)
          }
        }
        n234 = local read "Cookbook"() -> (w592:T13)
        n235 = local read "Motors"() -> (w589:bool)
        n236 = call "Run Cookbook.vi"("Cookbook"=w592, "Mod/Seq"="Mod/Seq", "Save to FITS?"="Save Data to FITS?", "limit max FPS to:"="limit max FPS to:", "Motors"=w589, "Error in"=w587, "Cameras in"=w568, "FITS Header In"=w590) -> ("Result"=w583:string, "FITS Path Out"=→"FITS Path from Last Recipe Acquiring Data":path, "Cameras out"=w567:refnum<class "Camera.lvclass">[], "Updated Header"=w579:T18, "Error out"=w586:errorcluster)  [unwired: 3 in]
        n237 = flat-sequence {
          tunnel: [w598] -> w562
          tunnel: w586 -> [w598]
          tunnel: [w597] -> w585
          frame #0 {
            n238 = Get Date/Time In Seconds() -> (seconds since 1Jan1904=w597:timestamp)
          }
        }
        n239 = Subtract(x=w585, y=w584) -> (x-y=w561:dbl)
        n240 = Greater Or Equal?(x=w561, y=60.0) -> (x >= y?=w559:bool)
        n241 = Format Date/Time String(time format string (%c)="%M:%S] ", seconds (now)=w561) -> (date/time string=w581:string)  [unwired: 1 in]
        n242 = case shown="True" w559 {
          frame False {
          }
          frame True {
            n243 = call "SCMP - Cbk end sound.vi"() -> ()  [unwired: 12 in]
          }
        }
        n244 = Concatenate Strings(w583, " [" ("string"), w581) -> (w596:string)
        n245 = call "SCMP - Write log v2.vi"("Error to log"=w562, "data"=w596) -> ("error out"=w595:errorcluster, "Last Log Entry"=w571:string)  [unwired: 7 in, 1 out]
        n246 = Concatenate Strings(w571, w570) -> (w572:string)
        n247 = Insert Into Array(array=w566, index=0, new element=Main_Program_States."Update UI" ("Beginning State")) -> (w565:T17[])
      }
      frame "Set Filter Wheel" {
        n248 = disable-structure shown="SCMP==COMP, Default" {
          disable-tunnel: w614 -> [w625 w632]
          disable-tunnel: [w624 w631] -> w613
          disable-tunnel: [w618 w626] -> w611
          disable-tunnel: [w622 w630] -> w607
          disable-tunnel: w608 -> [w623 w629]
          frame condition #0 {
            n249 = disable-structure shown="Disabled" {
              frame Disabled {
                # "old filter wheel vi"
                n250 = call "Optec IFW3 - Standalone.vi"() -> ()  [unwired: 11 in, 1 out]
              }
              frame Enabled {
              }
            }
            n251 = call "SCD - wavelenght.vi"("SCD Emission Line Filter"="Emission Line Filters") -> ("Numeric"=w619:dbl)  [unwired: 10 in]
            n252 = call "Optec IFW3 - Set Position with Error Handling.vi"("error in"=w625, "Emission Line Filter"="Emission Line Filters", "Filter Wheel Selector"=T23."Emission Line Filters") -> ("error out"=w618:errorcluster, "Actual Position (1-9)"=w624:i32)  [unwired: 6 in, 1 out]
            n253 = Bundle By Name(cluster=w623, "SCD Emission Line Filter"="Emission Line Filters", "Wavelength (nm)"=w619) -> (w622:T18)
          }
          frame condition #1 (active) {
            n254 = call "COMP - wavelenght.vi"("COMP-S Andover Filter Wheel"="Andover Filter Wheel") -> ("Wavelength (nm)"=w627:dbl)  [unwired: 10 in]
            n255 = call "CoMP-S Mechanism - FW.vi"("error in (no error)"=w632, "Emission Line Filters [530.3 nm]"="Andover Filter Wheel", "Filter Wheel Selector"=T23."Emission Line Filters") -> ("error out"=w626:errorcluster, "Position"=w631:i32)  [unwired: 5 in, 2 out]
            n256 = Bundle By Name(cluster=w629, "COMP-S Andover Filter Wheel"="Andover Filter Wheel", "Wavelength (nm)"=w627) -> (w630:T18)
          }
        }
        n257 = Number To Decimal String(number=w613) -> (decimal integer string=w609:string)  [unwired: 1 in]
        n258 = Concatenate Strings("Updated Filter Wheel to position:" ("data"), "\t", w609) -> (w610:string)
        n259 = call "SCMP - Write log v2.vi"("Error to log"=w611, "data"=w610) -> ("error out"=w612:errorcluster, "Last Log Entry"=w616:string)  [unwired: 7 in, 1 out]
        n260 = Insert Into Array(array=w604, index=0, new element=Main_Program_States."Update UI" ("Next State")) -> (w603:T17[])
      }
      frame "Set Calibration Wheel" {
        n261 = disable-structure shown="SCMP==COMP, Default" {
          disable-tunnel: w645 -> [w652 w659]
          disable-tunnel: [w657 w663] -> w643
          disable-tunnel: [w656 w662] -> w641
          disable-tunnel: [w654 w661] -> w639
          disable-tunnel: w640 -> [w655 w660]
          frame condition #0 {
            n262 = disable-structure shown="Disabled" {
              frame Disabled {
                # "old filter wheel vi"
                n263 = call "Optec IFW3 - Standalone.vi"() -> ()  [unwired: 11 in, 1 out]
              }
              frame Enabled {
              }
            }
            n264 = Bundle By Name(cluster=w655, "SCD Calibration Optics"="Calibration Optics") -> (w654:T18)
            n265 = call "Optec IFW3 - Set Position with Error Handling.vi"("error in"=w652, "SCD Calibration Optics"="Calibration Optics", "Filter Wheel Selector"=T23."Calibration Polarizers") -> ("error out"=w657:errorcluster, "Actual Position (1-9)"=w656:i32)  [unwired: 6 in, 1 out]
          }
          frame condition #1 (active) {
            n266 = Bundle By Name(cluster=w660, "COMP-S Calibration Wheel"="Calibration Wheel") -> (w661:T18)
            n267 = call "CoMP-S Mechanism - FW.vi"("error in (no error)"=w659, "Calibration Polarizer Filters [Dark]"="Calibration Wheel", "Filter Wheel Selector"=T23."Calibration Polarizers") -> ("error out"=w663:errorcluster, "Position"=w662:i32)  [unwired: 5 in, 2 out]
          }
        }
        n268 = Number To Decimal String(number=w641) -> (decimal integer string=w649:string)  [unwired: 1 in]
        n269 = Concatenate Strings("Updated Calibration Wheel to position:" ("data"), "\t", w649) -> (w642:string)
        n270 = call "SCMP - Write log v2.vi"("Error to log"=w643, "data"=w642) -> ("error out"=w644:errorcluster, "Last Log Entry"=w647:string)  [unwired: 7 in, 1 out]
        n271 = Insert Into Array(array=w637, index=0, new element=Main_Program_States."Wait for Event" ("Next State")) -> (w636:T17[])
      }
      frame "AISAS Motors on/off" {
        n272 = Unbundle By Name(w672) -> ("Peripherals"=w674:T16)
        n273 = Select(t="on" ("data"), s="Motors", f="off" ("data")) -> (s? t:f=w679:string)
        n274 = call "Mech on_off.vi"("Peripherals in"=w674, "error in (no error)"=w677, "Motors"="Motors") -> ("error out"=w684:errorcluster, "auto off log"=w670:string, "Peripherals out"=w673:T16)  [unwired: 6 in]
        n275 = Bundle By Name(cluster=w672, "Peripherals"=w673) -> (w671:T18)
        n276 = Concatenate Strings("AISAS Motors " ("data"), w679, w670) -> (w678:string)
        n277 = call "SCMP - Write log v2.vi"("Error to log"=w684, "data"=w678) -> ("error out"=w676:errorcluster, "Last Log Entry"=w675:string)  [unwired: 7 in, 1 out]
        n278 = Insert Into Array(array=w668, index=0, new element=Main_Program_States."Wait for Event" ("Next State")) -> (w667:T17[])
      }
      frame "AISAS Move" {
        n279 = Unbundle By Name(w707) -> ("Peripherals.AISAS Mech.lvclass"=w705:refnum<class "AISAS Mech.lvclass">)
        n280 = call "Move.vi"("error in (no error)"=w706, "AISAS Mech in"=w705) -> ("error out"=w704:errorcluster, "AISAS Mech out"=w702:refnum<class "AISAS Mech.lvclass">)  [unwired: 7 in, 1 out]
        n281 = Bundle By Name(cluster=w707, "Peripherals.AISAS Mech.lvclass"=w702) -> (w696:T18)
        n282 = call "Read value.vi"("error in (no error)"=w704, "AISAS Mech in"=w702) -> ("error out"=w703:errorcluster, "Rotation"=w695:T11, "Focus"=w694:T5, "Diffuser"=w698:T10, "Motor"=w697:T22, "Value (String)"=w699:string, "Motor (String)"=w701:string)  [unwired: 3 in]
        n283 = Concatenate Strings("AISAS " ("data"), w701, " set to: " ("data"), w699) -> (w709:string)
        n284 = call "SCMP - Write log v2.vi"("Error to log"=w703, "data"=w709) -> ("error out"=w693:errorcluster, "Last Log Entry"=w708:string)  [unwired: 7 in, 1 out]
        n285 = case shown="\"Rotation\"" w697 {
          tunnel: w698 -> [w713 _ _]
          tunnel: w696 -> [w714 w717 w720]
          tunnel: w694 -> [_ w716 _]
          tunnel: w695 -> [_ _ w719]
          tunnel: [w712 w715 w718] -> w691
          frame "Diffuser " {
            n286 = Bundle By Name(cluster=w714, "Light Shapping Diffuser"=w713) -> (w712:T18)
          }
          frame "Focus" {
            n287 = Bundle By Name(cluster=w717, "Objective Lens Position (mm)"=w716) -> (w715:T18)
          }
          frame "Rotation" {
            n288 = Bundle By Name(cluster=w720, "FOV Rotation (deg)"=w719) -> (w718:T18)
          }
        }
        n289 = call "SCMP write init xml.vi"("error in (no error)"=w693, "FITS Header In"=w691) -> ("error out"=w692:errorcluster)  [unwired: 8 in, 1 out]
        n290 = Insert Into Array(array=w689, index=0, new element=Main_Program_States."Update UI" ("Next State")) -> (w688:T17[])
      }
      frame "Change Camera Stage Position" {
        n291 = Build Array("PI cam1 (mm)", "PI cam2 (mm)", "PI cam3 (mm)") -> (w733:T3[])
        n292 = call "SCMP - Control PI Stage Position2.vi"("error in"=w738, "Absolute (F) or \nRelative (T) Move"=FALSE ("Absolute (F) or \nRelative (T) Move"), "set values"=w733) -> ("error out"=w734:errorcluster, "PI set?"=w730:bool, "Position"=w731:dbl[])  [unwired: 6 in]
        n293 = case shown="True" w730 {
          tunnel: ["" w754] -> w739
          tunnel: w729 -> [w741 w753]
          tunnel: [w741 w752] -> w736
          tunnel: [w742 w751] -> w735
          tunnel: w734 -> [w742 w744]
          tunnel: w731 -> [_ w743]
          frame False {
          }
          frame True {
            n294 = Bundle By Name(cluster=w753, "Camera PI (mm)"=w743) -> (w752:T18)
            n295 = Number To Fractional String(number=w743, width (-)=i16 6, precision (6)=i16 2) -> (F-format string=w749:string[])  [unwired: 1 in]
            n296 = Concatenate Strings("Camera Moved to Positon:" ("Recent Log"), w749, "\n" ("string")) -> (w748:string)
            n297 = call "SCMP - Write log v2.vi"("Error to log"=w744, "data"=w748) -> ("error out"=w751:errorcluster, "Last Log Entry"=w754:string)  [unwired: 7 in, 1 out]
          }
        }
        n298 = Insert Into Array(array=w724, index=0, new element=Main_Program_States."Update UI" ("Next State")) -> (w723:T17[])
      }
      frame "Change Camera Exposure" {
        n299 = Unbundle By Name(w769) -> ("Cameras"=w771:T12)
        n300 = call "Cams select.vi"("Cameras"=w771, "Cameras in"=w765) -> ("Cams selection"=w770:refnum<class "Camera.lvclass">[], "Cams indx"=w767:i32)  [unwired: 8 in]
        n301 = for {
          shift-right: [w779] -> w760
          shift-left: w774 -> [w781]
          tunnel: [w777] -> w763
          tunnel: w770 -> [w780] mode=indexing
          tunnel: "Exposure (s)" -> [w778]
          tunnel: [w776] -> w766 mode=indexing
          n302 = call-dynamic "Set exp.vi"("error in (no error)"=w781, "Exposure (s)"=w778, "Camera in"=w780) -> ("error out"=w779:errorcluster, "Exposure (s) out"=w777:dbl, "Camera out"=w776:refnum<class "Camera.lvclass">)  [unwired: 6 in]
        }
        n303 = Replace Array Subset(array=w765, new element=w766, index=w767) -> (w764:refnum<class "Camera.lvclass">[])
        n304 = Format Into String(format string="Camera Exposure Changed to %.2ps " ("data"), error in=w760, w763) -> (resulting string=w761:string, error out=w759:errorcluster)  [unwired: 1 in]
        n305 = call "SCMP - Write log v2.vi"("Error to log"=w759, "data"=w761) -> ("error out"=w773:errorcluster, "Last Log Entry"=w775:string)  [unwired: 7 in, 1 out]
        n306 = Insert Into Array(array=w758, index=0, new element=Main_Program_States."Update UI" ("Beginning State")) -> (w757:T17[])
      }
      frame "Set Camera AOI" {
        n307 = Unbundle By Name(w786) -> ("Cameras"=w795:T12)
        n308 = call "Cams select.vi"("Cameras"=w795, "Cameras in"=w793) -> ("Cams selection"=w789:refnum<class "Camera.lvclass">[], "Cams indx"=w794:i32)  [unwired: 8 in]
        n309 = for {
          shift-right: [w805] -> w791
          shift-left: w792 -> [w806]
          tunnel: w789 -> [w804] mode=indexing
          tunnel: [w803] -> w788 mode=indexing
          tunnel: "Binning" -> [w802]
          n310 = call-dynamic "Set binning.vi"("error in (no error)"=w806, "Binning"=w802, "Camera in"=w804) -> ("error out"=w805:errorcluster, "Camera out"=w803:refnum<class "Camera.lvclass">)  [unwired: 7 in]
        }
        n311 = Replace Array Subset(array=w793, new element=w788, index=w794) -> (w790:refnum<class "Camera.lvclass">[])
        n312 = property on="Binning" class="Enum (strict)"() -> ("RingText.Text"=w797:string)  [unwired: 2 in, 2 out]
        n313 = Concatenate Strings("Set Camera Binning: " ("Recent Log"), w797) -> (w800:string)
        n314 = call "SCMP - Write log v2.vi"("Error to log"=w791, "data"=w800) -> ("error out"=w798:errorcluster, "Last Log Entry"=w799:string)  [unwired: 7 in, 1 out]
        n315 = Insert Into Array(array=w785, index=0, new element=Main_Program_States."Update UI" ("Beginning State")) -> (w784:T17[])
      }
      frame "Andor Adv Settings" {
        n316 = call "Cams select.vi"("Cameras"=Cameras_select."Andor", "Cameras in"=w812) -> ("Cams selection"=w815:refnum<class "Camera.lvclass">[], "Cams indx"=w813:i32)  [unwired: 8 in]
        n317 = for {
          tunnel: w815 -> [w834] mode=indexing
          tunnel: [w833] -> w820 mode=indexing
          n318 = call-dynamic "Read Cam info.vi"("Camera in"=w834) -> ("Handle"=w833:i32)  [unwired: 5 in, 9 out]
        }
        n319 = Index Array(array=w820) -> (element #1=w819:i32, element #2=w818:i32)  [unwired: 2 in]
        n320 = call-by-ref "SCMP Andor setupdialog.vi"(error in=w824, "Handle 2"=w818, "Handle"=w819) -> (error out=w817:errorcluster)  [unwired: 10 in, 2 out]
        n321 = for {
          tunnel: w815 -> [w832] mode=indexing
          shift-right: [w828] -> w816
          shift-left: w817 -> [w829]
          tunnel: [w825] -> w814 mode=indexing
          n322 = To More Specific Class(target class=refnum<class "Andor.lvclass"> refnum ("Andor.lvclass"), reference=w832) -> (specific class reference=w831:refnum<class "Andor.lvclass">)  [unwired: 1 in, 1 out]
          n323 = call "Andor Neo check.vi"("error in"=w829, "Andor.lvclass"=w831) -> ("error out"=w828:errorcluster, "Andor.lvclass out"=w827:refnum<class "Andor.lvclass">)  [unwired: 5 in, 3 out]
          n324 = To More Generic Class(target class=refnum<class "Camera.lvclass"> refnum ("Camera.lvclass"), reference=w827) -> (generic class reference=w825:refnum<class "Camera.lvclass">)
        }
        n325 = Replace Array Subset(array=w812, new element=w814, index=w813) -> (w811:refnum<class "Camera.lvclass">[])
        n326 = Insert Into Array(array=w809, index=0, new element=Main_Program_States."Update UI" ("Beginning State")) -> (w808:T17[])
      }
      frame "Stop" {
        n327 = Unbundle By Name(w841) -> ("Peripherals.PI Stages"=w840:bool)
        n328 = global read "Global demo.vi" "demo"() -> (w844:bool)
        n329 = Not(x=w844) -> (.not. x?=w842:bool)
        n330 = Compound Arithmetic op=AND(w842, w838, w840) -> (w843:bool)
        n331 = case shown="True" w843 {
          tunnel: [FALSE w853] -> w845
          frame False {
          }
          frame True {
            n332 = Two Button Dialog(message="Set PI stages to parking position?", 1:"No" ("F button name (\"Cancel\")"), 2:"Yes" ("T button name (\"OK\")")) -> (T button?=w853:bool)
          }
        }
        n333 = case shown="True" w845 {
          tunnel: w848 -> [w858 w867]
          tunnel: [w858 w866] -> w847
          tunnel: ["Main Loop Terminated" ("data") w863] -> w846
          frame False {
          }
          frame True {
            w864 = "\n" ("string")
            n334 = disable-structure shown="SCMP==COMP, Default" {
              disable-tunnel: [w874 w875] -> w868
              frame condition #0 (active) {
                n335 = global read "Globals.vi" "comp parking pos"() -> (w874:dbl[])
              }
              frame condition #1 {
                n336 = global read "Globals.vi" "scd parking pos"() -> (w875:dbl[])
              }
            }
            n337 = call "SCMP - Control PI Stage Position2.vi"("error in"=w867, "Absolute (F) or \nRelative (T) Move"=FALSE ("Absolute (F) or \nRelative (T) Move"), "set values"=w868) -> ("error out"=w866:errorcluster, "Position"=w862:dbl[])  [unwired: 6 in, 1 out]
            n338 = Index Array(array=w862) -> (element #1=w859:dbl, element #2=w860:dbl, element #3=w861:dbl)  [unwired: 3 in]
            n339 = Number To Fractional String(number=w862, width (-)=i16 6, precision (6)=i16 2) -> (F-format string=w872:string[])  [unwired: 1 in]
            n340 = local write "PI cam1 (mm)"(w859) -> ()
            n341 = local write "PI cam2 (mm)"(w860) -> ()
            n342 = local write "PI cam3 (mm)"(w861) -> ()
            n343 = Concatenate Strings("Camera Moved to Positon:" ("Recent Log"), w872, w864, "Main Loop Terminated" ("data"), w864) -> (w863:string)
          }
        }
        n344 = call "SCMP - Write log v2.vi"("Error to log"=w847, "data"=w846) -> ("error out"=w849:errorcluster, "Last Log Entry"=w851:string)  [unwired: 7 in, 1 out]
        n345 = Build Array(Main_Program_States."Stop" ("Next State")) -> (w835:T17[])
      }
    }
    "FITS Header" <- w92
    n346 = Not(x=w91) -> (.not. x?=→"Main Loop":bool)
    n347 = Concatenate Strings(w99, w100) -> (w98:string)
    "Latest Actions" <- w98
    n348 = local write "Main Loop Error"(w94) -> ()
    n349 = call <vilib>:"General Error Handler.vi"("error in (no error)"=w94) -> ("error out"=w95:errorcluster)  [unwired: 10 in, 4 out]
    n350 = call <vilib>:"Clear Errors.vi"("error in (no error)"=w95) -> ("error out"=w97:errorcluster)  [unwired: 5 in, 1 out]
  }
  n351 = while {
    shift-right: [w880] -> _
    shift-left: w3 -> [w877]
    tunnel: [w887] -> w32
    shift-right: [w884] -> _
    shift-left: 0.0 ("Time Target (s)") -> [w882]
    shift-right: [w878] -> w17
    shift-left: w18 -> [w881]
    stop <- w886 stop-if-true
    n352 = call "Elapsed Time"("Time Target (s)"=w882, "error in (no error)"=w877) -> ("Time has Elapsed"=w885:bool, "error out"=w876:errorcluster)  [unwired: 10 in, 6 out]
    n353 = case shown="True" w885 {
      tunnel: w876 -> [w889 w895]
      tunnel: [w889 w894] -> w879
      tunnel: w882 -> [w890 _]
      tunnel: [w890 w893] -> w884
      tunnel: w881 -> [w888 w892]
      tunnel: [w888 w891] -> w878
      frame False {
      }
      frame True {
        w893 = 10.0  # Log cadence time [s]
        n354 = stacked-sequence {
          frame #0 {
            n355 = local write "Log Loop"(FALSE ("Log Loop")) -> ()
            n356 = Wait (ms)(milliseconds to wait=u32 200) -> ()  [unwired: 1 out]
          }
          frame #1 {
            n357 = local write "Log Loop"(TRUE ("Log Loop")) -> ()
          }
        }
        n358 = case shown="True" "Enable Data Logging" {
          tunnel: w895 -> [w901 w913]
          tunnel: [w901 w908] -> w894
          tunnel: w892 -> [w900 w904]
          tunnel: [w900 w910] -> w891
          frame False {
          }
          frame True {
            n359 = call "Read Zone Temps v2.vi"("Peripherals"=w904, "error in"=w913) -> ("error out"=w903:errorcluster, "Air Temp [C]"=w902:dbl, "Camera Body [C]"=w914:sgl, "Pre-Filter Temp [C}"=w911:sgl, "Peripherals out"=w909:T16)  [unwired: 5 in]
            "Air around Camera [C]" <- w914
            "Air around \nprefilter wheel [C]" <- w911
            "Air around Lyot Filter [C]" <- w902
            n360 = call "ILX Status.vi"("Peripherals in"=w909, "error in"=w903) -> ("error out"=w912:errorcluster, "Temperature"=w915:dbl, "Peripherals out"=w910:T16)  [unwired: 4 in, 3 out]
            "Lyot Filter Temp [C]" <- w915
            n361 = local read "Camera 1 Temp [C}"() -> (w907:dbl)
            n362 = Build Array(w915, w911, w914, w902, w907) -> (w906:dbl[])
            n363 = disable-structure shown="SCMP==COMP, Default" {
              disable-tunnel: w906 -> [w917 w919]
              disable-tunnel: [w916 w919] -> w905
              frame condition #0 (active) {
                n364 = local read "Camera 2 Temp [C}"() -> (w918:dbl)
                n365 = Build Array (concatenate)(w917, w918) -> (w916:dbl[])
              }
              frame condition #1 {
              }
            }
            n366 = call "SCMP - Write Eng Data v2.vi"("error in"=w912, "Temp Data"=w905) -> ("error out"=w908:errorcluster)  [unwired: 6 in, 3 out]
            "Eng Data Error" <- w908
          }
        }
      }
    }
    n367 = local read "Main Loop"() -> (w887:bool)
    n368 = Wait (ms)(milliseconds to wait=u32 100) -> ()  [unwired: 1 out]
    n369 = Not(x=w887) -> (.not. x?=w886:bool)
    n370 = call <vilib>:"Clear Errors.vi"("error in (no error)"=w879) -> ("error out"=w880:errorcluster)  [unwired: 5 in, 1 out]
  }
  "Log Loop" <- w32
  n371 = Unbundle By Name(w17) -> ("Zone temp ref"=w8:variant)
  n372 = call "Close all.vi"("error in (no error)"=w30, "Cameras"=w5) -> ("error out"=w33:errorcluster)  [unwired: 9 in]
  n373 = disable-structure shown="Disabled" {
    frame Disabled {
      (unwired) string[] ["Cookbook Stopped"] ("[user-defined descriptions]")
      w921 = T24 2 items=["no dialog", "OK message", "continue or stop message", "OK message + warnings", "continue/stop + warnings"] ("type of dialog (OK msg:1)")
      n374 = call <vilib>:"General Error Handler.vi"("[user-defined codes]"=i32[] [5000], "type of dialog (OK msg:1)"=w921) -> ("[user-defined descriptions]"=w923:string[])  [unwired: 8 in, 5 out]
      n375 = One Button Dialog(message="Please Enter \nAn Observer\nAnd A Comment") -> ()  [unwired: 1 in, 1 out]
    }
    frame Enabled {
    }
  }
  n376 = Variant To Data(type=refnum<k24> refnum ("ILabVIEW In"), Variant=w8) -> (data=w7:refnum<k24>)  [unwired: 1 in, 1 out]
  n377 = Not A Number/Path/Refnum?(number/path/refnum=w7) -> (NaN/Path/Refnum?=w6:bool)
  n378 = case shown="False" w6 {
    tunnel: [w925 errorcluster {"status"=FALSE, "code"=0, "source"=""} ("error out")] -> w29
    tunnel: w7 -> [w924 _]
    frame False {
      n379 = call "Std_Bus_Close_System.vi"("ILabVIEW In"=w924) -> ("error out"=w925:errorcluster)  [unwired: 1 in, 17 out]
    }
    frame True {
    }
  }
  n380 = Merge Errors(w33, w29) -> (w25:errorcluster)
  n381 = Unbundle By Name(w25) -> ("status"=w26:bool)
  n382 = call "SCMP - Write log v2.vi"("Error to log"=w25, "data"="Program Ended") -> ("error out"=→"Main Loop Error":errorcluster)  [unwired: 7 in, 2 out]
  n383 = And(x=FALSE, y=w26) -> (x .and. y?=→"Program":bool)
  "Instrument" <- w10
